vi "Conus_USB.vi"() -> ()   [LabVIEW 2017]
doc: "Conus USB - Versió bàsica de Conus / Sols adquisició i informe"
uses:
  Instance           2 17Saved   Conus_USB .vi
  Instance           1 17Saved   Conus_USB .vi
  Instance           4 17Saved   Conus_USB .vi
  <vilib>/DAQmx/write.llb/DAQmx Write (Digital 1D Bool NChan 1Samp 1Line).vi
  <vilib>/DAQmx/read.llb/DAQmx Read (Digital 1D Bool NChan 1Samp 1Line).vi
  Control 1.ctl
panel:
  out "Array":bool[](array[boolean])
  out "data":bool[](array[boolean])
  out "Fent_Rep":bool
  out "Booleans":refnum<vi>[](array[refnum])
  in  "Rep. Fetes":u8 caption="N. Rep."
  in  "Salir":bool caption="Sortir"
  in  "EtiquetaTipusParo":string caption="String"
  in  "Etiqueta Velocitats":string caption="String"
  out "appended array":refnum<vi>[](array[refnum])
  out "MissatgesUsuari":string[](array[string])
  out "Caselles":refnum<vi>[](array[refnum])
  out "StringsEstatMáquina":string[](array[string])
  in  "Rep. A Fer":sgl caption="N. Rep." format="%#_1g"
  out "ParoDefor":bool caption="ParoRotura"
  out "ParoDeforFet":bool caption="ParoProcessat"
  out "ParoCargaFet":bool caption="ParoProcessat"
  out "ParoCarga":bool caption="ParoProcessat"
  in  "CaptadorD":u16(ring) caption="Unidades" items=["Deformació", "Extensòmetre"]
  in  "FinalEnsayo":bool caption="Final prova"
  in  "ActivaParoCarga":bool caption="ActivaParoDefor"
  in  "ValorParoCarga":sgl caption="Força" min=0 format="%#.3f"
  in  "ActivaParoDefor":bool
  in  "ActivaParoRotura":T1
  in  "ValorParoDesplazamiento":sgl caption="Deformació" min=0 format="%#.3f"
  in  "ValorParoRotura":sgl caption="Ruptura (%)" min=0 format="%#_3f"
  out "Ensayo activo":bool caption="Prova en marxa"
  out "ArraiMostresxProva":dbl[](array[numeric])
  out "NMostres":dbl
  in  "BtEliminarUltima":bool=TRUE caption="Eliminar última prova"
  out "Estado ensayo:":string caption="Estat assaig:"
  out "CodiAturada":u32
  out "ViuMotor":bool
  out "MotorBipolar":bool
  out "Baixar":bool
  out "Pujar":bool
  out "PrimerCaptador":i32
  out "rings":refnum<vi>[](array[refnum])
  in  "IndexUnitatsD":u8
  in  "IndexUnitatsF":u8
  in  "IndexCaptadorD":u8
  in  "IndexCaptadorF":u8
  out "EtiquetesRegistre":string[](array[string])
  out "start":bool
  out "Active_motor":bool
  in  "Inici x Boto":bool
  out "ExtenPoten":bool caption="Extensòmetre Pot."
  out "ValorSenseTara":dbl
  in  "VelocitatMàxima":dbl
  in  "PerCentPrecarga":sgl=0.5 caption="Precàrrega (%)"
  in  "Precarga":bool
  in  "BtMaxF":bool
  in  "CaptadorF":u16(ring) caption="Unidades" items=["1000 kg"=11, "No presente"=23]
  in  "UnidadesF":u16(ring) caption="Unidades" items=["kg", "N"]
  in  "BtTaraF":bool caption="TARA"
  out "Fuerza":sgl caption="Força" format="%.1f"
  out "Nº Tests":u8 caption="Tests:"
  out "Sobrecarga":bool caption="Sobrecàrrega"
  out "Paro Manual":bool caption="Aturada Manual"
  out "FCI":bool
  out "FCS":bool
  in  "ResoExten":i8(ring) caption="Resolució Extensometre" items=["0.1", "0.2", "0.5", "0.01", "0.02", "0.05", "0.001", "0.002", "0.005"]
  out "PrecargaOn":bool
  in  "ValorPrecarga":dbl caption="Precarga (%)"
  out "Calibratge D":dbl[](array[numeric])
  out "Extensometre":bool
  in  "UnidadesD":u16(ring) caption="Unidades" items=["mm", "inch"]
  in  "BtTaraD":bool caption="TARA"
  out "Deformacion":sgl caption="Deformació" format="%.1f"
  out "Celula_0":u8
  in  "Células":u8(ring) caption="Célula 1" items=["0.5 kg", "1 Kg", "2 Kg", "5 kg", "10 kg", "20 kg", "50 kg", "100 kg", "200 kg", "300 kg", "500 kg", "1000 kg", "2000 kg", "5000 kg", "10000 kg", "20000 kg", "30000 kg", "P-20 kg", "P-200 kg", "P-500 kg", "P-5000 kg", "P-20000 kg", "P-50 bar", "No presente"]
  in  "UnidadesF_C2":u16(ring) caption="Unidades" items=["kg"]
  in  "UnidadesF_C1":u16(ring) caption="Unidades" items=["kg", "N"]
  out "ArraiUnitats":cluster{"String":string, "Value":u16}[](array[cluster])=[{"String"="kg", "Value"=0}, {"String"="N", "Value"=1}, {"String"="g", "Value"=2}, {"String"="daN", "Value"=3}, {"String"="cN", "Value"=4}, {"String"="KN", "Value"=5}, {"String"="lb", "Value"=6}]
  in  "UnitatsF":u8[](array[numeric])
  in  "Velocidad Retorno":sgl caption="Retorn" min=0 max=500 step=1 format="%#.1f"
  in  "Velocidad Ensayo":sgl caption="Assaig" min=0 step=1
  out "ValorSobrecargaC2":dbl
  out "Valor de control sobrecarga":dbl
  out "Calibratge":dbl[](array[numeric])
  in  "ParaAssaig":bool
  out "ParoProcessat":bool
  out "Salidas_mando":T2={"HI_down"=TRUE, " LO_down"=TRUE, "HI_up"=TRUE, "*"=TRUE, " LO_up"=TRUE, " start"=TRUE, " Ensayo_down"=TRUE, " Ensayo_up"=TRUE}
  out "VelocitatMotor":dbl min=0.0 max=500.0 step=1.0
  out "TempsLectura":u32=150
  out "Maxim":sgl
  in  "Inhibicio":bool
  in  "Ensayonuevo":bool caption="Assaig Nou"
  in  "Guardar":bool caption="Informe"
  in  "Iniciar / Finalizar":bool=TRUE caption="Finalitzar prova"
  out "TablaFinal":dbl[][](array[numeric])
  out "Tabla":dbl[][](array[numeric])
  in  "Columna":i32
  out "Paro Emergencia":bool
  out "ParoRotura":bool
  out "AssaigMM":bool
  out "DSenseTara":sgl caption="Fuerza - N"
  out "FactorsUnitatsPendents_D":dbl[](array[numeric])
  out "ConversioUnitatsD":dbl[](array[numeric])=[1.0, 9.8756, 1000.0, 0.98]
  in  "DadesAdquirides":dbl[](array[numeric]) format="%#_8g"
  out "FactorsUnitatsPendents_F":dbl[](array[numeric])
  in  "LedAssaig":bool
  out "BaixarMM":bool
  out "PujarMM":bool
  in  "TaraD":sgl
  in  "ValMax":bool
  out "FSenseTara":sgl caption="Fuerza - N"
  in  "TaraF":sgl
  out "Password":string
  out "ValorSobrecargaC1":dbl
  out "ConversioUnitatsF":dbl[](array[numeric])=[1.0, 9.8756, 2.2]
  out "Pendents":dbl[](array[numeric]) format="%#_8g"
  in  "Procesa datos":bool
  in  "Stop":bool=TRUE
  in  "First time":bool
  out "?":cluster{"Y":dbl[], "Y":dbl[]}[](graph)
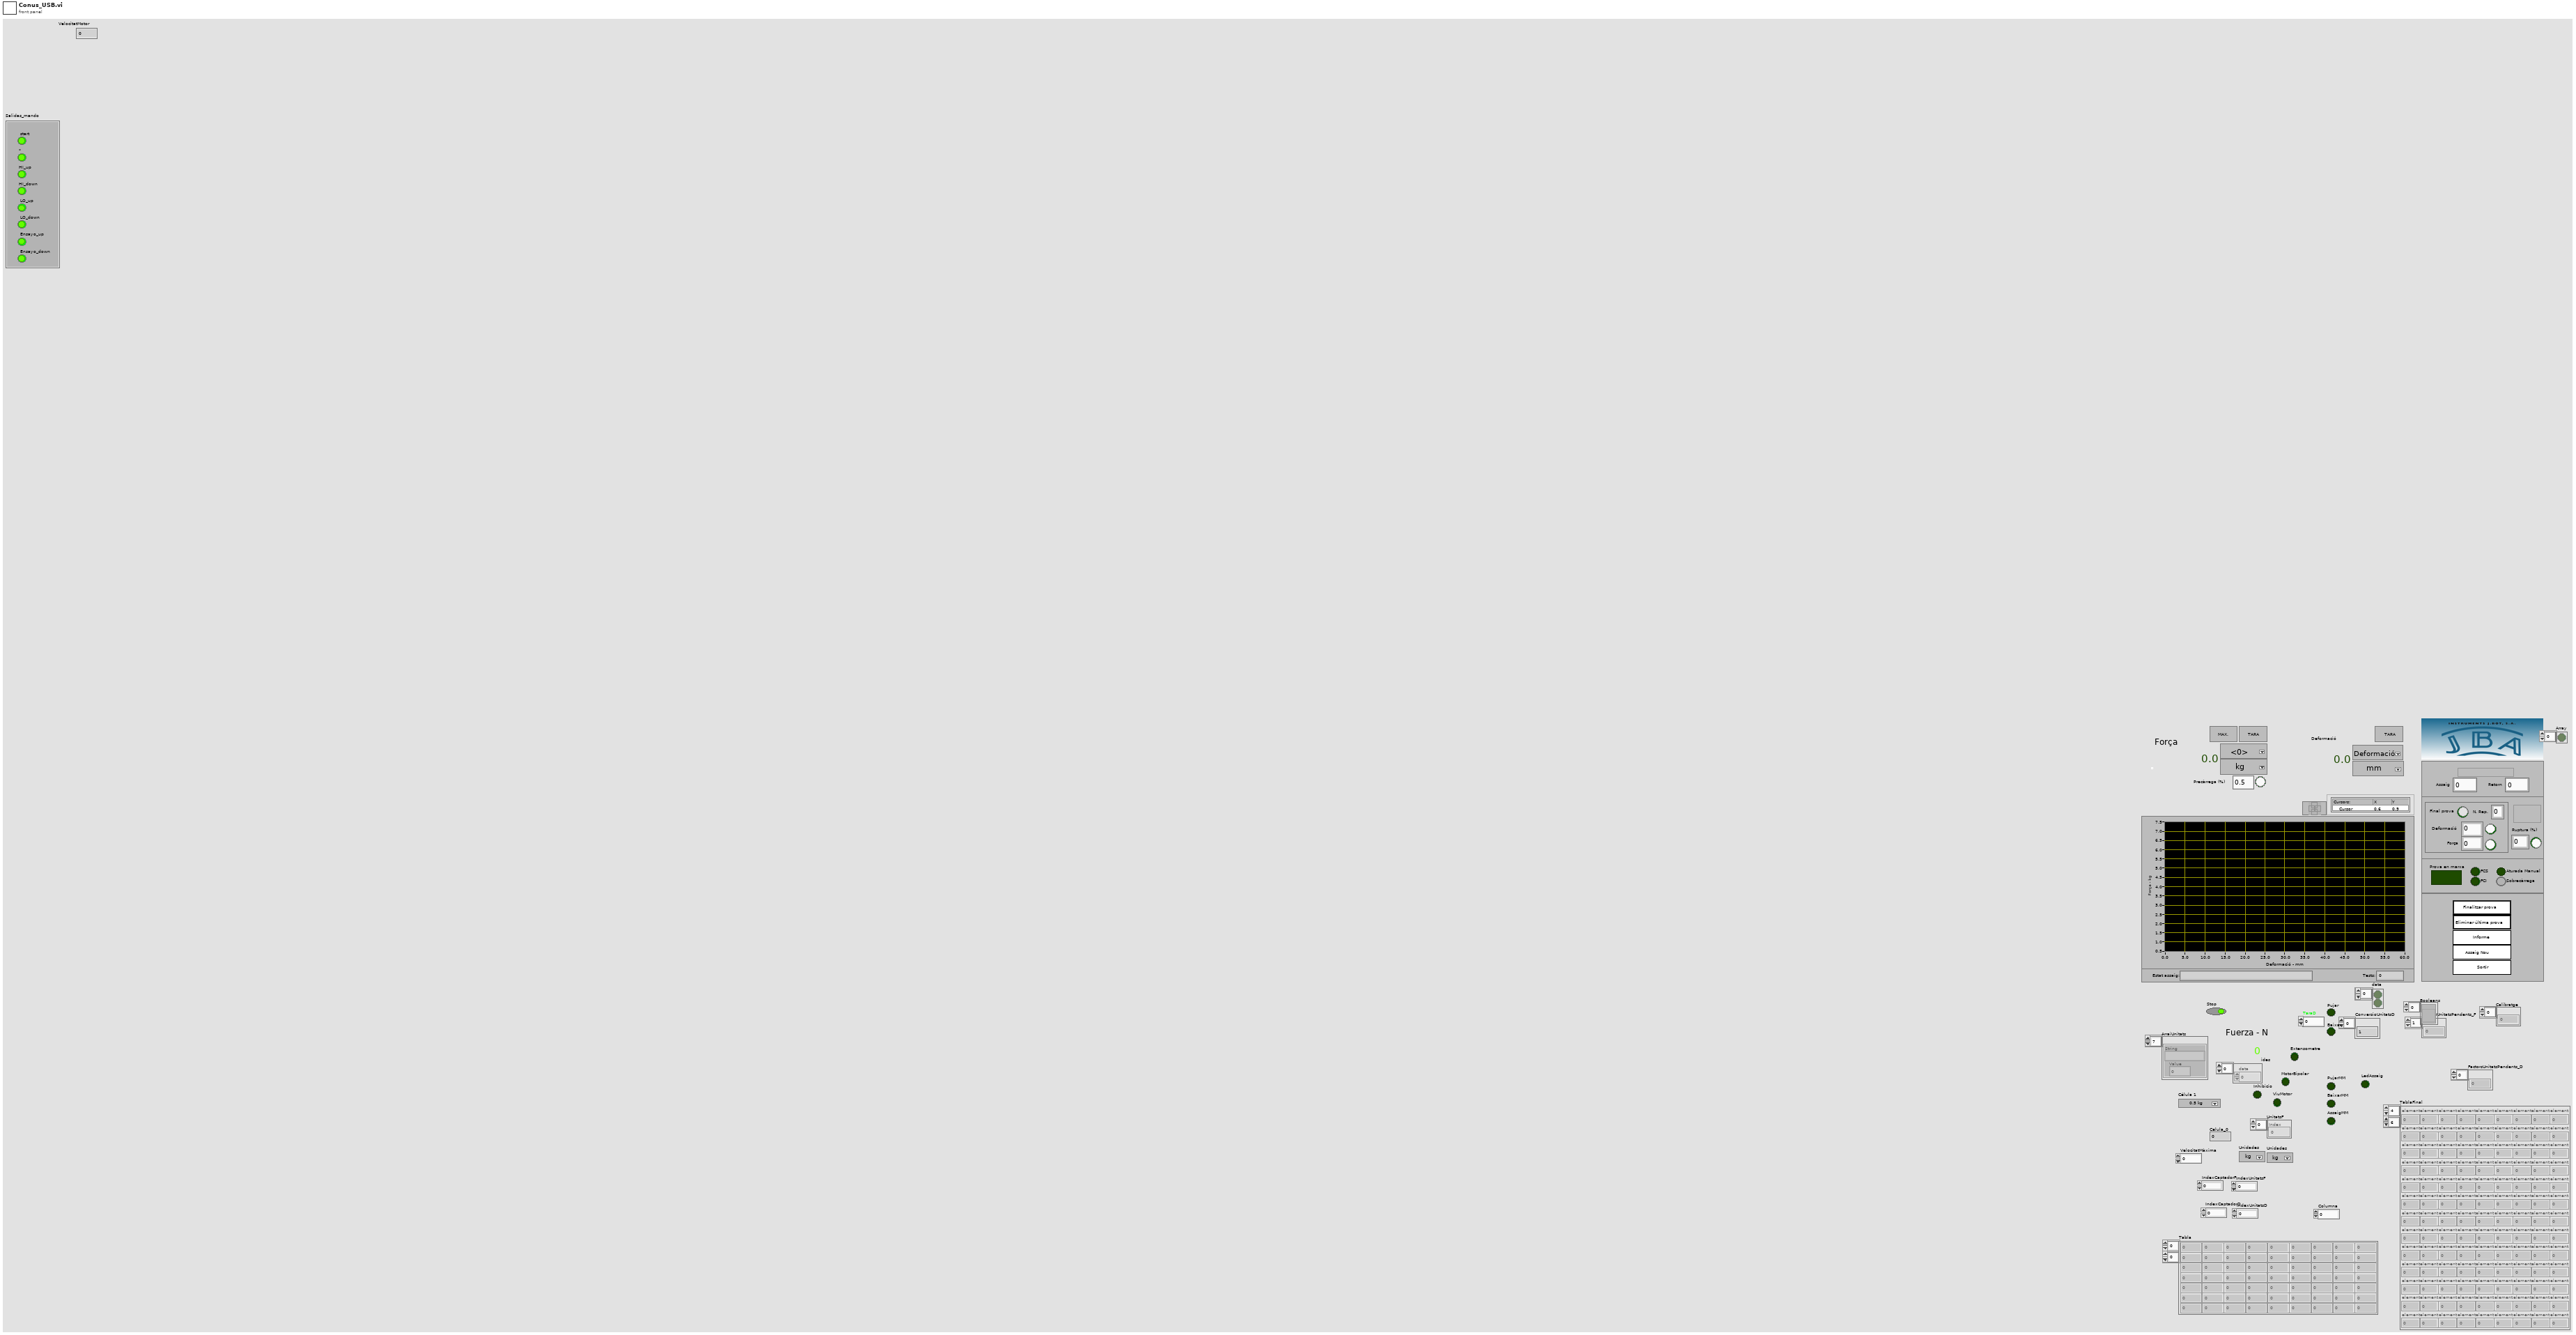
[diagram p1: front panel]
types:
  T1 = typedef "Control 1.ctl" = bool
  T2 = cluster{"HI_down":bool, " LO_down":bool, "HI_up":bool, "*":bool, " LO_up":bool, " start":bool, " Ensayo_down":bool, " Ensayo_up":bool}
  T3 = cluster{"HI_down":bool, "LO_down":bool, "HI_up":bool, "*":bool, "LO_up":bool, "start":bool, "Ensayo_down":bool, "Ensayo_up":bool}
  T4 = typedef "LVStringsAndValuesArrayTypeDef_U8.ctl" = cluster{"String":string, "Value":u8}[]
  T5 = cluster{"Boolean":bool, "element":bool, "Boolean":bool, "Boolean":bool}
  T6 = typedef "LVStringsAndValuesArrayTypeDef_U16.ctl" = cluster{"String":string, "Value":u16}[]
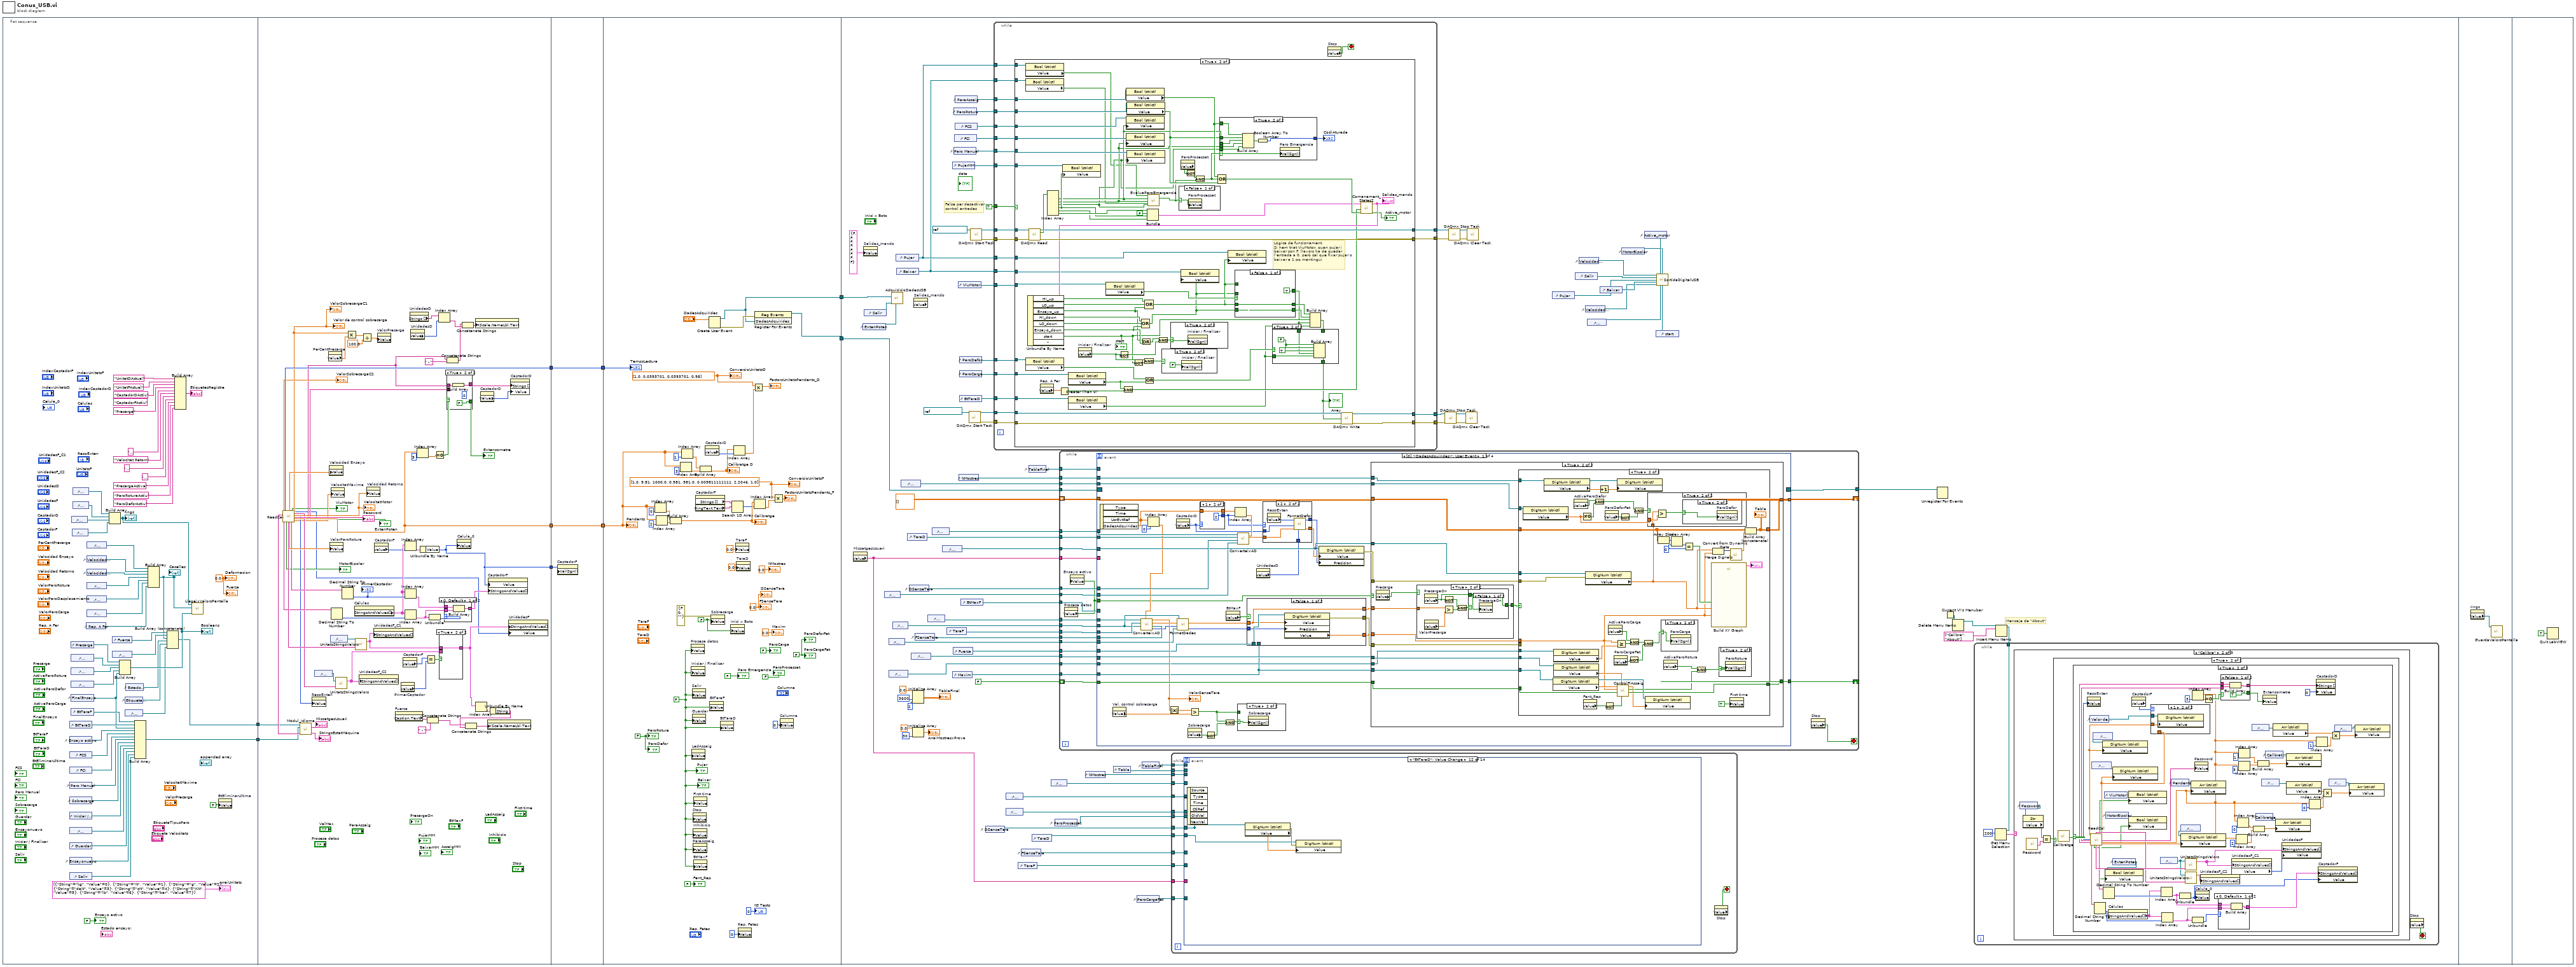
[diagram p0: block diagram]
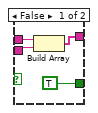
[diagram p3: hidden frame]
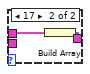
[diagram p4: hidden frame]
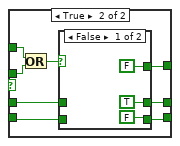
[diagram p7: hidden frame]
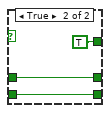
[diagram p8: hidden frame]
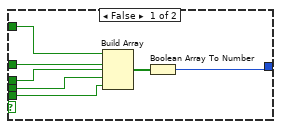
[diagram p11: hidden frame]
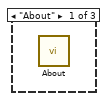
[diagram p13: hidden frame]
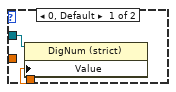
[diagram p16: hidden frame]
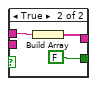
[diagram p17: hidden frame]
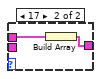
[diagram p18: hidden frame]
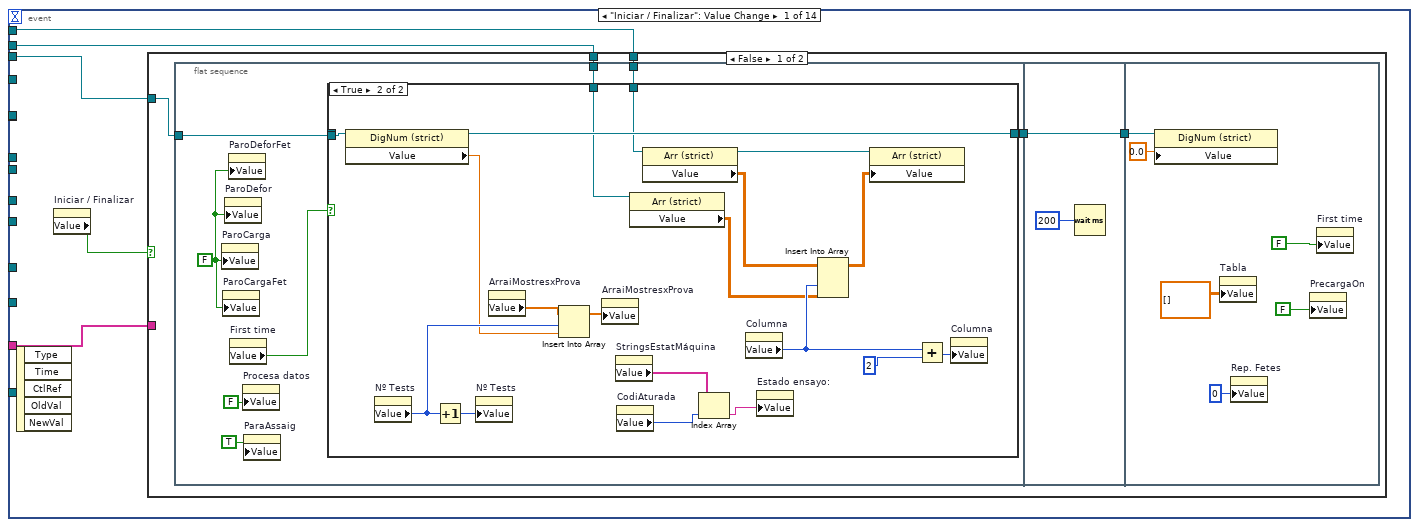
[diagram p20: hidden frame]
diagram:
  n1 = flat-sequence {
    tunnel: [w19] -> w2
    tunnel: [w18] -> w1
    tunnel: [w111] -> w9
    tunnel: [w126] -> w8
    tunnel: [w74] -> w3
    tunnel: w2 -> [w66]
    tunnel: w1 -> [w68]
    tunnel: w9 -> [w145]
    tunnel: [w145] -> w7
    tunnel: w8 -> [w144]
    tunnel: [w144] -> w6
    tunnel: w3 -> [w143]
    tunnel: w7 -> [w164]
    tunnel: [w183] -> w5
    tunnel: [w175] -> w4
    tunnel: w6 -> [w174]
    tunnel: w5 -> [w267]
    tunnel: w4 -> [w249]
    frame #0 {
      w12 = sgl 0.0 ("Deformacion")
      (unwired) "CaptadorFActiu" ("value")
      n2 = control-ref of="BtTaraD"() -> (w39:refnum<vi>)
      n3 = control-ref of="Ensayo activo"() -> (w37:refnum<vi>)
      n4 = control-ref of="FCS"() -> (w36:refnum<vi>)
      n5 = control-ref of="FCI"() -> (w35:refnum<vi>)
      n6 = control-ref of="Paro Manual"() -> (w34:refnum<vi>)
      n7 = control-ref of="Sobrecarga"() -> (w33:refnum<vi>)
      n8 = control-ref of="Iniciar / Finalizar"() -> (w32:refnum<vi>)
      n9 = control-ref of="BtEliminarUltima"() -> (w31:refnum<vi>)
      n10 = control-ref of="Guardar"() -> (w17:refnum<vi>)
      n11 = control-ref of="Ensayonuevo"() -> (w30:refnum<vi>)
      n12 = control-ref of="Salir"() -> (w29:refnum<vi>)
      n13 = control-ref of="Precarga"() -> (w50:refnum<vi>)
      n14 = control-ref of="ActivaParoRotura"() -> (w49:refnum<vi>)
      n15 = control-ref of="ActivaParoDefor"() -> (w48:refnum<vi>)
      n16 = control-ref of="ActivaParoCarga"() -> (w42:refnum<vi>)
      n17 = control-ref of="FinalEnsayo"() -> (w38:refnum<vi>)
      n18 = control-ref of="BtTaraF"() -> (w40:refnum<vi>)
      n19 = control-ref of="CaptadorD"() -> (w45:refnum<vi>)
      n20 = control-ref of="CaptadorF"() -> (w44:refnum<vi>)
      n21 = control-ref of="UnidadesD"() -> (w47:refnum<vi>)
      n22 = control-ref of="UnidadesF"() -> (w46:refnum<vi>)
      n23 = control-ref of="Rep. A Fer"() -> (w10:refnum<vi>)
      n24 = control-ref of="PerCentPrecarga"() -> (w27:refnum<vi>)
      n25 = control-ref of="Velocidad Ensayo"() -> (w26:refnum<vi>)
      n26 = control-ref of="Velocidad Retorno"() -> (w51:refnum<vi>)
      n27 = control-ref of="ValorParoRotura"() -> (w25:refnum<vi>)
      n28 = control-ref of="ValorParoDesplazamiento"() -> (w24:refnum<vi>)
      n29 = control-ref of="ValorParoCarga"() -> (w23:refnum<vi>)
      n30 = Build Array(w47, w46, w45, w44) -> (w43:refnum<vi>[])
      "rings" <- w43
      n31 = control-ref of="Fuerza"() -> (w22:refnum<vi>)
      n32 = control-ref of="Deformacion"() -> (w21:refnum<vi>)
      n33 = Build Array(w50, w49, w48, w42, w38) -> (w28:refnum<vi>[])
      "Booleans" <- w28
      n34 = control-ref of="Etiqueta Velocitats"() -> (w14:refnum<vi>)
      n35 = control-ref of="EtiquetaTipusParo"() -> (w13:refnum<vi>)
      n36 = control-ref of="Estado ensayo:"() -> (w15:refnum<vi>)
      n37 = Build Array(w40, w39, w38, w37, w36, w35, w34, w33, w32, w31, w17, w30, w29) -> (w19:refnum<vi>[])
      n38 = Build Array(w27, w26, w51, w25, w24, w23, w10) -> (w16:refnum<vi>[])
      "Caselles" <- w16
      n39 = Build Array (concatenate)(w22, w21, w16, w15, w14, w13) -> (w18:refnum<vi>[])
      n40 = Build Array("UnitatDActual" ("value"), "UnitatFActual" ("value"), "CaptadorDActiu" ("value"), "Precarga" ("value"), "Velocitat" ("value"), "Velocitat Retorn" ("value"), "Rotura" ("value"), "Desplazamiento" ("value"), "PrecargaActiva" ("value"), "ParoRoturaActiu" ("value"), "ParoDeforActiu" ("value")) -> (→"EtiquetesRegistre":string[])
      n41 = call "LlegeixValorsPantalla.vi"("rings"=w43, "Caselles 2"=w16, "Booleans"=w28) -> ()  [unwired: 8 in]
      n42 = property on="BtEliminarUltima" class="Bool (strict)"("Value"=FALSE ("BtEliminarUltima")) -> ()  [unwired: 2 in, 2 out]
      "Ensayo activo" <- FALSE ("Ensayo activo")
      "Fuerza" <- w12
      "Deformacion" <- w12
      "ArraiUnitats" <- cluster{"String":string, "Value":u16}[] [{"String"="kg", "Value"=0}, {"String"="N", "Value"=1}, {"String"="g", "Value"=2}, {"String"="daN", "Value"=3}, {"String"="cN", "Value"=4}, {"String"="KN", "Value"=5}, {"String"="lb", "Value"=6}, {"String"="bar", "Value"=7}] ("Strings And Values [] 2")
    }
    frame #1 {
      n43 = call "ReadCal.vi"() -> ("SobrecargaC2"=→"ValorSobrecargaC2":dbl, "ResoExten"=w103:i8, "TextExtensometre"=w108:string, "TextDeformacio"=w67:string, "SegonCaptador"=w118:string, "TempsLectura"=w126:u16, "Idioma"=w70:string, "MotorBipolar"=→"MotorBipolar":bool, "UnitatsC2"=w119:string, "UnitatsC1"=w120:string, "Velocitat"=w127:dbl, "ParoRotura"=w128:dbl, "V. Retorn"=w123:dbl, "PrimerCaptador"=w116:string, "ViuMotor"=→"ViuMotor":bool, "ExtenPoten"=→"ExtenPoten":bool, "Unidades"=w64:u8, "SobrecargaC1"=w104:dbl, "Password"=→"Password":string, "Pendents"=w111:dbl[], "VelocitatMàxima"=w100:dbl)  [unwired: 4 in, 3 out]
      "VelocitatMotor" <- w123
      "ValorSobrecargaC1" <- w104
      "Valor de control sobrecarga" <- w104
      n44 = call "Módul_Idioma.vi"("Idioma"=w70, "Array"=w66, "Caselles"=w68) -> ("TextosEstatMaquina"=→"StringsEstatMáquina":string[], "MissatgesUsuari"=→"MissatgesUsuari":string[])  [unwired: 7 in]
      n45 = property on="ResoExten" class="Ring (strict)"("Value"=w103) -> ()  [unwired: 2 in, 2 out]
      n46 = control-ref of="ArraiUnitats"() -> (w121:refnum<vi>)
      n47 = property on="PerCentPrecarga" class="DigNum (strict)"() -> ("Value"=w94:sgl)  [unwired: 2 in, 2 out]
      n48 = property on="Velocidad Ensayo" class="DigNum (strict)"("Value"=w127) -> ()  [unwired: 2 in, 2 out]
      n49 = property on="ValorParoRotura" class="DigNum (strict)"("Value"=w128) -> ()  [unwired: 2 in, 2 out]
      n50 = control-ref of="ArraiUnitats"() -> (w122:refnum<vi>)
      n51 = property on="VelocitatMàxima" class="DigNum (strict)"("Value"=w100) -> ()  [unwired: 2 in, 2 out]
      n52 = Decimal String To Number(string=w118) -> (number=w117:i32)  [unwired: 2 in, 1 out]
      n53 = call "UnitatsStringsValors.vi"("UnitatsC1"=w119, "Arr Refnum"=w121) -> ("Array 2"=w84:cluster{"String":string, "Value":u16}[])  [unwired: 1 out]
      n54 = Decimal String To Number(string=w116) -> (number=w115:i32)  [unwired: 2 in, 1 out]
      "PrimerCaptador" <- w115
      n55 = Multiply(x=w104, y=w94) -> (x*y=w106:dbl)
      n56 = property on="Células" class="Ring (strict)"() -> ("StringsAndValues[]"=w91:T4)  [unwired: 2 in, 2 out]
      n57 = call "UnitatsStringsValors.vi"("UnitatsC1"=w120, "Arr Refnum"=w122) -> ("Array 2"=w85:cluster{"String":string, "Value":u16}[])  [unwired: 1 out]
      n58 = property on="UnidadesF_C2" class="Ring (strict)"("StringsAndValues[]"=w84) -> ()  [unwired: 2 in, 2 out]
      n59 = Divide(x=w106, y=100.0) -> (x/y=w101:dbl)
      n60 = property on="Velocidad Retorno" class="DigNum (strict)"("Value"=w123) -> ()  [unwired: 2 in, 2 out]
      n61 = property on="UnidadesF_C1" class="Ring (strict)"("StringsAndValues[]"=w85) -> ()  [unwired: 2 in, 2 out]
      n62 = property on="CaptadorF" class="Ring (strict)"() -> ("Value"=w89:u16)  [unwired: 2 in, 2 out]
      n63 = property on="ValorPrecarga" class="DigNum (strict)"("Value"=w101) -> ()  [unwired: 2 in, 2 out]
      n64 = property on="Fuerza" class="DigNum (strict)"() -> ("Caption.Text"=w97:string)  [unwired: 2 in, 2 out]
      n65 = property on="PrimerCaptador" class="DigNum (strict)"() -> ("Value"=w86:i32)  [unwired: 2 in, 2 out]
      n66 = property on="CaptadorF" class="Ring (strict)"() -> ("Value"=w87:u16)  [unwired: 2 in, 2 out]
      n67 = Index Array(array=w91, index=w89) -> (element=w90:cluster{"String":string, "Value":u8})
      n68 = Index Array(array=w91, index=w115) -> (element=w93:cluster{"String":string, "Value":u8})
      n69 = Index Array(array=w91, index=w117) -> (element=w113:cluster{"String":string, "Value":u8})
      n70 = property on="UnidadesD" class="Ring (strict)"() -> ("Strings []"=w79:string[])  [unwired: 2 in, 2 out]
      n71 = property on="UnidadesD" class="Ring (strict)"() -> ("Value"=w78:u16)  [unwired: 2 in, 2 out]
      n72 = Index Array(array=w111, index=3) -> (element=w109:dbl)
      n73 = Unbundle By Name(w90) -> ("Value"=w74:u8)
      n74 = Equal?(x=w87, y=w86) -> (x = y?=w88:bool)
      n75 = Concatenate Strings(w97, " - ") -> (w96:string)
      n76 = Unbundle(w113) -> ("Value"=w114:u8)  [unwired: 1 out]
      n77 = Equal To 0?(x=w109) -> (x = 0?=w112:bool)
      n78 = Index Array(array=w79, index=w78) -> (element=w77:string)
      n79 = case shown="True" w88 {
        tunnel: w85 -> [_ w130]
        tunnel: [w129 w130] -> w65
        tunnel: w84 -> [w129 _]
        frame False {
        }
        frame True {
        }
      }
      n80 = case shown="0, Default" w114 {
        tunnel: w93 -> [w140 w141]
        tunnel: w113 -> [w139 _]
        tunnel: [w138 w142] -> w92
        frame 0, Default {
          n81 = Build Array(w140, w139) -> (w138:cluster{"String":string, "Value":u8}[])
        }
        frame 17 {
          n82 = Build Array(w141) -> (w142:cluster{"String":string, "Value":u8}[])
        }
      }
      n83 = Concatenate Strings(w67, " - ") -> (w75:string)
      n84 = case shown="True" w112 {
        tunnel: w108 -> [w134 _]
        tunnel: [w133 w135] -> w80
        tunnel: [TRUE ("Extensometre") FALSE ("Extensometre")] -> w107
        tunnel: w67 -> [w131 w136]
        frame False {
          n85 = Build Array(w131, w134) -> (w133:string[])
        }
        frame True {
          (unwired) 0 ("index")
          n86 = Build Array(w136) -> (w135:string[])
        }
      }
      "Extensometre" <- w107
      n87 = property on="Celula_0" class="DigNum (strict)"("Value"=w74) -> ()  [unwired: 2 in, 2 out]
      n88 = Concatenate Strings(w75, w77) -> (w95:string)
      n89 = property class="XYGraph (strict)"("XScale.NameLbl.Text"=w95) -> ()  [unwired: 2 in, 2 out]
      n90 = Index Array(array=w65) -> (element=w82:cluster{"String":string, "Value":u16})  [unwired: 1 in]
      n91 = property on="CaptadorD" class="Ring (strict)"() -> ("Value"=w81:u16)  [unwired: 2 in, 2 out]
      n92 = property on="CaptadorF" class="Ring (strict)"("Value"=w74, "StringsAndValues[]"=w92) -> ()  [unwired: 2 in, 2 out]
      n93 = Unbundle By Name(w82) -> ("String"=w83:string)
      n94 = Concatenate Strings(w96, w83) -> (w102:string)
      n95 = property class="XYGraph (strict)"("YScale.NameLbl.Text"=w102) -> ()  [unwired: 2 in, 2 out]
      n96 = property on="UnidadesF" class="Ring (strict)"("StringsAndValues[]"=w65, "Value"=w64) -> ()  [unwired: 2 in, 2 out]
      n97 = property on="CaptadorD" class="Ring (strict)"("Strings []"=w80, "Value"=w81) -> ()  [unwired: 2 in, 2 out]
    }
    frame #2 {
      n98 = property on="CaptadorF" class="Ring (strict)"("Val(Sgnl)"=w143) -> ()  [unwired: 2 in, 2 out]
    }
    frame #3 {
      w149 = FALSE ("ParoCargaFet")
      w148 = FALSE ("ParoRotura")
      w162 = dbl[] [1.0, 0.0393701, 0.0393701, 0.98]
      w177 = sgl 0.0 ("FSenseTara")
      w185 = dbl[] [1.0, 9.81, 1000.0, 0.981, 981.0, 0.009811111111, 2.2046, 1.0]
      w156 = FALSE ("Sobrecarga")
      w152 = FALSE ("Iniciar / Finalizar")
      n99 = Index Array(array=w164, index=0) -> (element=w170:dbl)
      n100 = Index Array(array=w164, index=2) -> (element=w171:dbl)
      n101 = Build Array(w170, w171) -> (w169:dbl[])
      "Calibratge" <- w169
      n102 = Index Array(array=w164, index=3) -> (element=w165:dbl)
      n103 = Index Array(array=w164, index=1) -> (element=w163:dbl)
      n104 = property on="Procesa datos" class="Bool (strict)"("Value"=w152) -> ()  [unwired: 2 in, 2 out]
      n105 = property on="Iniciar / Finalizar" class="Bool (strict)"("Value"=w152) -> ()  [unwired: 2 in, 2 out]
      n106 = property on="LedAssaig" class="Bool (strict)"("Value"=w152) -> ()  [unwired: 2 in, 2 out]
      n107 = property on="Salir" class="Bool (strict)"("Value"=w152) -> ()  [unwired: 2 in, 2 out]
      n108 = property on="Guardar" class="Bool (strict)"("Value"=w152) -> ()  [unwired: 2 in, 2 out]
      n109 = property on="Stop" class="Bool (strict)"("Value"=w152) -> ()  [unwired: 2 in, 2 out]
      n110 = property on="Inhibicio" class="Bool (strict)"("Value"=w152) -> ()  [unwired: 2 in, 2 out]
      n111 = property on="ParaAssaig" class="Bool (strict)"("Value"=w152) -> ()  [unwired: 2 in, 2 out]
      n112 = property on="First time" class="Bool (strict)"("Value"=w152) -> ()  [unwired: 2 in, 2 out]
      n113 = property on="BtMaxF" class="Bool (strict)"("Value"=w152) -> ()  [unwired: 2 in, 2 out]
      n114 = property on="CaptadorF" class="Ring (strict)"() -> ("Strings []"=w155:string[], "RingText.Text"=w154:string)  [unwired: 2 in, 2 out]
      n115 = Build Array(w163, w165) -> (w160:dbl[])
      "Calibratge D" <- w160
      n116 = property on="CaptadorD" class="Ring (strict)"() -> ("Value"=w161:u16)  [unwired: 2 in, 2 out]
      n117 = Create User Event(user event datatype="DadesAdquirides") -> (user event=w175:refnum<user-event>, error out=w182:errorcluster)  [unwired: 1 in]
      n118 = property on="BtTaraF" class="Bool (strict)"("Value"=w152) -> ()  [unwired: 2 in, 2 out]
      n119 = property on="Sobrecarga" class="Bool (strict)"(error in=errorcluster {"status"=FALSE, "code"=0, "source"=""} ("error in (no error)"), "Value"=w156) -> ()  [unwired: 1 in, 2 out]
      n120 = property on="BtTaraD" class="Bool (strict)"("Value"=w152) -> ()  [unwired: 2 in, 2 out]
      n121 = property on="Inici x Boto" class="Bool (strict)"("Value"=w156) -> ()  [unwired: 2 in, 2 out]
      n122 = Search 1D Array(1D array=w155, element=w154) -> (index of element=w153:i32)  [unwired: 1 in]
      n123 = Index Array(array=w160, index=w161) -> (element=w159:dbl)
      n124 = property on="TaraF" class="DigNum (strict)"("Value"=sgl 0.0 ("Tara")) -> ()  [unwired: 2 in, 2 out]
      n125 = property on="TaraD" class="DigNum (strict)"("Value"=sgl 0.0 ("TaraD")) -> ()  [unwired: 2 in, 2 out]
      n126 = property on="Rep. Fetes" class="DigNum (strict)"("Value"=u8 0 ("Rep. Fetes")) -> ()  [unwired: 2 in, 2 out]
      n127 = Multiply(x=w162, y=w159) -> (x*y=→"FactorsUnitatsPendents_D":dbl[])
      n128 = Index Array(array=w169, index=w153) -> (element=w168:dbl)
      n129 = register-events(error in=w182, w175) -> (reference out=w183:refnum<event-registration>)  [unwired: 1 in, 1 out]
      n130 = Multiply(x=w185, y=w168) -> (x*y=→"FactorsUnitatsPendents_F":dbl[])
      n131 = property on="Columna" class="DigNum (strict)"("Value"=0 ("Columna")) -> ()  [unwired: 2 in, 2 out]
      "Pendents" <- w164
      "ConversioUnitatsF" <- w185
      "FSenseTara" <- w177
      "ConversioUnitatsD" <- w162
      "DSenseTara" <- w177
      "ParoRotura" <- w148
      "Paro Emergencia" <- FALSE ("Paro Emergencia")
      "Maxim" <- sgl 0.0 ("Maxim")
      "TempsLectura" <- w174
      "ParoProcessat" <- FALSE ("ParoProcessat")
      "Nº Tests" <- u8 0 ("Nº Tests")
      "Pujar" <- w152
      "Baixar" <- w152
      "NMostres" <- 0.0 ("NMostres")
      "ParoCarga" <- FALSE ("ValorCargaFet")
      "ParoCargaFet" <- w149
      "ParoDeforFet" <- w149
      "ParoDefor" <- w148
      "Fent_Rep" <- FALSE ("Fent_Rep")
    }
    frame #4 {
      # "False per desactivar\ncontrol entrades"
      # "Mensaje de \"About\""
      n132 = property on="MissatgesUsuari" class="Arr (strict)"() -> ("Value"=w195:string[])  [unwired: 2 in, 2 out]
      n133 = control-ref of="ExtenPoten"() -> (w216:refnum<vi>)
      n134 = property on="Salidas_mando" class="Clust (strict)"("Value"=T3 {"HI_down"=FALSE, "LO_down"=FALSE, "HI_up"=FALSE, "*"=FALSE, "LO_up"=FALSE, "start"=FALSE, "Ensayo_down"=FALSE, "Ensayo_up"=FALSE} ("Salidas_mando")) -> ()  [unwired: 2 in, 2 out]
      n135 = control-ref of="Salir"() -> (w250:refnum<vi>)
      n136 = control-ref of="UnidadesD"() -> (w260:refnum<vi>)
      n137 = control-ref of="ValorParoCarga"() -> (w200:refnum<vi>)
      n138 = control-ref of="CaptadorF"() -> (w225:refnum<vi>)
      n139 = call "AdquisicioDadesUSB.vi"(6:w216, "Stop"=w250, 10:w249) -> ()  [unwired: 9 in]
      n140 = control-ref of="UnidadesF"() -> (w259:refnum<vi>)
      n141 = control-ref of="Pujar"() -> (w206:refnum<vi>)
      n142 = control-ref of="Baixar"() -> (w205:refnum<vi>)
      n143 = control-ref of="ValorParoDesplazamiento"() -> (w221:refnum<vi>)
      n144 = control-ref of="TaraD"() -> (w263:refnum<vi>)
      n145 = control-ref of="DSenseTara"() -> (w264:refnum<vi>)
      n146 = control-ref of="ValorParoRotura"() -> (w256:refnum<vi>)
      n147 = Initialize Array(0.0 ("element"), 3600 ("dimension size"), 2 ("dimension size")) -> (→"TablaFinal":dbl[][])
      n148 = Initialize Array(0.0 ("element"), 30 ("dimension size")) -> (→"ArraiMostresxProva":dbl[])
      n149 = property on="Salidas_mando" class="Clust (strict)" props=["Value"]() -> ()  [unwired: 2 in, 3 out]
      n150 = control-ref of="FSenseTara"() -> (w269:refnum<vi>)
      n151 = control-ref of="FactorsUnitatsPendents_F"() -> (w268:refnum<vi>)
      n152 = control-ref of="FactorsUnitatsPendents_D"() -> (w266:refnum<vi>)
      n153 = control-ref of="Deformacion"() -> (w265:refnum<vi>)
      n154 = control-ref of="TaraF"() -> (w270:refnum<vi>)
      n155 = control-ref of="PujarMM"() -> (w208:refnum<vi>)
      n156 = control-ref of="Maxim"() -> (w248:refnum<vi>)
      n157 = control-ref of="Fuerza"() -> (w218:refnum<vi>)
      n158 = control-ref of="Paro Manual"() -> (w229:refnum<vi>)
      n159 = control-ref of="ParoRotura"() -> (w228:refnum<vi>)
      n160 = control-ref of="FCI"() -> (w230:refnum<vi>)
      n161 = control-ref of="ParaAssaig"() -> (w227:refnum<vi>)
      n162 = control-ref of="FCS"() -> (w231:refnum<vi>)
      n163 = control-ref of="ViuMotor"() -> (w209:refnum<vi>)
      n164 = control-ref of="NMostres"() -> (w201:refnum<vi>)
      n165 = control-ref of="ParoDefor"() -> (w198:refnum<vi>)
      n166 = control-ref of="ParoCarga"() -> (w199:refnum<vi>)
      n167 = control-ref of="BtTaraD"() -> (w193:refnum<vi>)
      n168 = control-ref of="BtMaxF"() -> (w223:refnum<vi>)
      n169 = call <vilib>:"DAQmx Start Task.vi"("task/channels in"=refnum<k21> "USBDigitalOut") -> ("task out"=w237:refnum<k21>, "error out"=w236:errorcluster)  [unwired: 13 in]
      n170 = call <vilib>:"DAQmx Start Task.vi"("task/channels in"=refnum<k21> "USBDigitalIn") -> ("task out"=w245:refnum<k21>, "error out"=w244:errorcluster)  [unwired: 13 in]
      n171 = control-ref of="DSenseTara"() -> (w261:refnum<vi>)
      n172 = while {
        tunnel: w245 -> [w298]
        tunnel: w244 -> [w297]
        tunnel: [w296] -> w240
        tunnel: [w295] -> w239
        tunnel: w237 -> [w294]
        tunnel: w236 -> [w293]
        tunnel: [w292] -> w233
        tunnel: [w291] -> w232
        tunnel: w231 -> [w290]
        tunnel: w230 -> [w289]
        tunnel: w229 -> [w288]
        tunnel: w228 -> [w287]
        tunnel: w227 -> [w286]
        tunnel: TRUE -> [w285]
        tunnel: w206 -> [w283]
        tunnel: w205 -> [w282]
        tunnel: w209 -> [w281]
        tunnel: w208 -> [w280]
        tunnel: w205 -> [w279]
        tunnel: w206 -> [w278]
        tunnel: w199 -> [w277]
        tunnel: w198 -> [w276]
        tunnel: w193 -> [w275]
        stop <- w284 stop-if-true
        n173 = case shown="True" w285 {
          tunnel: w298 -> [w302 w373]
          tunnel: w297 -> [w301 w372]
          tunnel: [w302 w371] -> w296
          tunnel: [w301 w370] -> w295
          tunnel: w294 -> [w300 w365]
          tunnel: w293 -> [w299 w364]
          tunnel: [w299 w363] -> w292
          tunnel: [w300 w362] -> w291
          tunnel: w290 -> [_ w359]
          tunnel: w289 -> [_ w358]
          tunnel: w288 -> [_ w357]
          tunnel: w287 -> [_ w350]
          tunnel: w286 -> [_ w347]
          tunnel: w283 -> [_ w340]
          tunnel: w282 -> [_ w339]
          tunnel: w281 -> [_ w337]
          tunnel: w280 -> [_ w327]
          tunnel: w279 -> [_ w324]
          tunnel: w278 -> [_ w323]
          tunnel: w277 -> [_ w314]
          tunnel: w276 -> [_ w313]
          tunnel: w275 -> [_ w305]
          frame False {
          }
          frame True {
            # "Lògica de funcionament.\nSi hem triat ViuMotor, quan pujar i baixar son F, llavors ha de quedar l'entrada a 0, però cal que fixar pujar o baixar a 1 pq mantingui"
            n174 = property class="Bool (strict)"(reference=w324) -> ("Value"=w317:bool)  [unwired: 1 in, 2 out]
            n175 = property class="Bool (strict)"(reference=w313) -> ("Value"=w312:bool)  [unwired: 1 in, 2 out]
            n176 = property class="Bool (strict)"(reference=w323) -> ("Value"=w318:bool)  [unwired: 1 in, 2 out]
            n177 = call-poly <vilib>:"DAQmx Read.vi"("task/channels in"=w373, "error in"=w372) -> ("task out"=w371:refnum<k21>, "data"=w331:bool[], "error out"=w370:errorcluster)  [unwired: 11 in]
            n178 = property on="Rep. A Fer" class="DigNum (strict)"() -> ("Value"=w309:sgl)  [unwired: 2 in, 2 out]
            n179 = Index Array(array=w331) -> (element #1=w321:bool, element #2=w320:bool, element #3=w319:bool, element #4=w325:bool, element #5=w326:bool, element #6=w361:bool)  [unwired: 6 in]
            n180 = Greater Than 0?(x=w309) -> (x > 0?=w307:bool)
            n181 = property class="Bool (strict)"(reference=w327, "Value"=w325) -> ()  [unwired: 1 in, 2 out]
            n182 = property class="Bool (strict)"(reference=w314) -> ("Value"=w308:bool)  [unwired: 1 in, 2 out]
            n183 = property class="Bool (strict)"(reference=w305) -> ("Value"=w303:bool)  [unwired: 1 in, 2 out]
            n184 = property on="Iniciar / Finalizar" class="Bool (strict)"() -> ("Value"=w344:bool)  [unwired: 2 in, 2 out]
            n185 = property class="Bool (strict)"(reference=w337) -> ("Value"=w336:bool)  [unwired: 1 in, 2 out]
            n186 = Not(x=w344) -> (.not. x?=w352:bool)
            n187 = And(x=w308, y=w307) -> (x .and. y?=w306:bool)
            n188 = property class="Bool (strict)"(reference=w347) -> ("Value"=w330:bool)  [unwired: 1 in, 2 out]
            n189 = property class="Bool (strict)"(reference=w359, "Value"=w321) -> ()  [unwired: 1 in, 2 out]
            n190 = property class="Bool (strict)"(reference=w358, "Value"=w320) -> ()  [unwired: 1 in, 2 out]
            n191 = property class="Bool (strict)"(reference=w350) -> ("Value"=w329:bool)  [unwired: 1 in, 2 out]
            n192 = property class="Bool (strict)"(reference=w357, "Value"=w319) -> ()  [unwired: 1 in, 2 out]
            n193 = Or(x=w312, y=w308) -> (x .or. y?=w311:bool)
            n194 = Bundle("Boolean"=w361, "element"=FALSE, "Boolean"=w325, "Boolean"=w326) -> (w310:T5)  [unwired: 1 in]
            n195 = call "EvaluaParoEmergencia.vi"("EsticPujant"=w318, "FCI"=w320, "FCS"=w321, "EsticBaixant"=w317, "ParoManual"=w319) -> ("Paro"=w322:bool)  [unwired: 10 in]
            n196 = case shown="False" w322 {
              selector: w322 -> [w398 _]
              frame False {
                n197 = property on="ParoProcessat" class="Bool (strict)"("Value"=w398) -> ()  [unwired: 2 in, 2 out]
              }
              frame True {
              }
            }
            n198 = property on="ParoProcessat" class="Bool (strict)"() -> ("Value"=w349:bool)  [unwired: 2 in, 2 out]
            n199 = Not(x=w349) -> (.not. x?=w348:bool)
            n200 = And(x=w348, y=w322) -> (x .and. y?=w346:bool)
            n201 = Compound Arithmetic op=OR(w330, w346, w329) -> (w345:bool)
            n202 = case shown="True" w346 {
              selector: w346 -> [_ w413]
              tunnel: w330 -> [w404 w412]
              tunnel: w329 -> [w403 w411]
              tunnel: w321 -> [w402 w410]
              tunnel: w320 -> [w401 w409]
              tunnel: w319 -> [w400 w408]
              tunnel: [w399 w406] -> w328
              frame False {
                n203 = Build Array(w404, w403, w402, w401, w400) -> (w405:bool[])
                n204 = Boolean Array To Number(Boolean array=w405) -> (number=w399:u32)
              }
              frame True {
                n205 = Build Array(w412, w411, w410, w409, w408) -> (w407:bool[])
                n206 = Boolean Array To Number(Boolean array=w407) -> (number=w406:u32)
                n207 = property on="Paro Emergencia" class="Bool (strict)"("Val(Sgnl)"=w413) -> ()  [unwired: 2 in, 2 out]
              }
            }
            "CodiAturada" <- w328
            n208 = call "Comanament_States2.vi"("Emergencia"=w345, "ReseUpDown"=w306, "Entradas_Botones"=w310) -> ("Active_motor"=→"Active_motor":bool, "Salidas_mando"=w351:T2)  [unwired: 5 in]
            "Salidas_mando" <- w351
            n209 = Unbundle By Name(w351) -> ("HI_up"=w369:bool, "LO_up"=w368:bool, "Ensayo_up"=w355:bool, "HI_down"=w367:bool, "LO_down"=w366:bool, "Ensayo_down"=w356:bool, "start"=w338:bool)  [unwired: 1 out]
            "start" <- w338
            n210 = Not(x=w338) -> (.not. x?=w343:bool)
            n211 = Or(x=w355, y=w356) -> (x .or. y?=w353:bool)
            n212 = Compound Arithmetic op=OR(w367, w366, w356) -> (w333:bool)
            n213 = And(x=w344, y=w343) -> (x .and. y?=w342:bool)
            n214 = Compound Arithmetic op=OR(w369, w368, w355) -> (w335:bool)
            n215 = And(x=w353, y=w352) -> (x .and. y?=w354:bool)
            n216 = case shown="True" w342 {
              frame False {
              }
              frame True {
                n217 = property on="Iniciar / Finalizar" class="Bool (strict)"("Val(Sgnl)"=FALSE ("Value (Signaling)")) -> ()  [unwired: 2 in, 2 out]
              }
            }
            n218 = case shown="True" w354 {
              selector: w354 -> [_ w414]
              frame False {
              }
              frame True {
                n219 = property on="Iniciar / Finalizar" class="Bool (strict)"("Val(Sgnl)"=w414) -> ()  [unwired: 2 in, 2 out]
              }
            }
            n220 = property class="Bool (strict)"(reference=w339, "Value"=w333) -> ()  [unwired: 1 in, 2 out]
            n221 = property class="Bool (strict)"(reference=w340, "Value"=w335) -> ()  [unwired: 1 in, 2 out]
            n222 = case shown="False" w336 {
              tunnel: w335 -> [_ w389]
              tunnel: w333 -> [_ w388]
              tunnel: [TRUE w383] -> w316
              tunnel: w335 -> [w381 w387]
              tunnel: [w381 w386] -> w334
              tunnel: w333 -> [w380 w385]
              tunnel: [w380 w384] -> w332
              frame False {
              }
              frame True {
                n223 = Or(x=w389, y=w388) -> (x .or. y?=w390:bool)
                n224 = case shown="False" w390 {
                  tunnel: w387 -> [_ w396]
                  tunnel: [TRUE w396] -> w386
                  tunnel: w385 -> [_ w395]
                  tunnel: [FALSE w395] -> w384
                  tunnel: [FALSE TRUE] -> w383
                  frame False {
                  }
                  frame True {
                  }
                }
              }
            }
            n225 = Build Array(w334, w332, w338, w316, w303) -> (w315:bool[])
            n226 = case shown="True" w311 {
              tunnel: w316 -> [_ w377]
              tunnel: [w374 w376] -> w304
              tunnel: w315 -> [w374 _]
              tunnel: w303 -> [_ w375]
              frame False {
              }
              frame True {
                w379 = FALSE
                n227 = Build Array(w379, w379, TRUE ("element"), w377, w375) -> (w376:bool[])
              }
            }
            "Array" <- w304
            n228 = call-poly <vilib>:"DAQmx Write.vi"("task/channels in"=w365, "data"=w304, "error in"=w364) -> ("task out"=w362:refnum<k21>, "error out"=w363:errorcluster)  [unwired: 10 in, 1 out]
          }
        }
        n229 = property on="Stop" class="Bool (strict)"() -> ("Value"=w284:bool)  [unwired: 2 in, 2 out]
      }
      n230 = control-ref of="FactorsUnitatsPendents_D"() -> (w220:refnum<vi>)
      n231 = control-ref of="FactorsUnitatsPendents_F"() -> (w226:refnum<vi>)
      n232 = control-ref of="TaraF"() -> (w257:refnum<vi>)
      n233 = control-ref of="FSenseTara"() -> (w258:refnum<vi>)
      n234 = control-ref of="TablaFinal"() -> (w189:refnum<vi>)
      n235 = control-ref of="TaraD"() -> (w262:refnum<vi>)
      n236 = control-ref of="CaptadorF"() -> (w224:refnum<vi>)
      n237 = control-ref of="ParoProcessat"() -> (w207:refnum<vi>)
      n238 = while {
        shift-right: [w833] -> _
        shift-left: dbl[][] [] -> [w832]
        tunnel: w268 -> [w831]
        tunnel: w270 -> [w820]
        tunnel: w218 -> [w830]
        tunnel: w269 -> [w829]
        tunnel: w267 -> [w827]
        tunnel: [w828] -> w222
        tunnel: w266 -> [w826]
        tunnel: w265 -> [w825]
        tunnel: w263 -> [w824]
        tunnel: w264 -> [w823]
        tunnel: w260 -> [w822]
        tunnel: w259 -> [w821]
        shift-right: [w819] -> _
        shift-left: FALSE ("ControlaCaigudaSortida") -> [w818]
        tunnel: w256 -> [w817]
        tunnel: w248 -> [w816]
        tunnel: w225 -> [w815]
        tunnel: w223 -> [w814]
        tunnel: w221 -> [w813]
        tunnel: w201 -> [w811]
        tunnel: w200 -> [w810]
        tunnel: w195 -> [w808]
        tunnel: w189 -> [w807]
        stop <- w812 stop-if-true
        n239 = property on="Procesa datos" class="Bool (strict)"() -> ("Value"=w809:bool)  [unwired: 2 in, 2 out]
        n240 = property on="Ensayo activo" class="Bool (strict)"("Value"=w809) -> ()  [unwired: 2 in, 2 out]
        n241 = event shown="[0] <DadesAdquirides>: User Event" {
          selector: w827 -> [_ _ _ _]
          dyn-events: [_ _ _ _] -> w828
          timeout: _ -> [_ _ _ _]
          tunnel: w832 -> [w881 w1003 w1064 _]
          tunnel: [w880 w1002 w1063 _] -> w833
          tunnel: w809 -> [w835 w1004 _ _]
          tunnel: w831 -> [w874 _ _ _]
          tunnel: w820 -> [w875 _ _ _]
          tunnel: w830 -> [w843 _ _ _]
          tunnel: w829 -> [w876 _ _ _]
          tunnel: w826 -> [w878 _ _ _]
          tunnel: w825 -> [w855 _ _ _]
          tunnel: w824 -> [w868 _ _ _]
          tunnel: w823 -> [w877 _ _ _]
          tunnel: w822 -> [w846 _ w1060 _]
          tunnel: w821 -> [w862 _ w1061 _]
          tunnel: [w873 _ _ _] -> w819
          tunnel: w818 -> [w872 _ _ _]
          tunnel: w817 -> [w871 _ w1058 _]
          tunnel: w816 -> [w857 _ _ _]
          tunnel: w815 -> [w861 _ _ _]
          tunnel: w814 -> [_ _ _ _]
          tunnel: w813 -> [w856 _ w1059 _]
          tunnel: w811 -> [w838 _ _ _]
          tunnel: w810 -> [w837 _ _ _]
          tunnel: w808 -> [_ w1001 _ w1087]
          tunnel: w807 -> [_ _ w1057 _]
          event User Event {
            n242 = event-data() -> ("DadesAdquirides"=w853:dbl[])  [unwired: 1 in, 3 out]
            n243 = property on="Val. control sobrecarga" class="DigNum (strict)"() -> ("Value"=w859:dbl)  [unwired: 2 in, 2 out]
            n244 = Index Array(array=w853, index=0) -> (element=w836:dbl)
            n245 = call "ConverteixAD.vi"("ValorSenseTara"=w876, "ValorAdquirid"=w836, "Unitats"=w862, "Tara"=w875, "FactorsUnitatsPendents"=w874) -> ("Escala"=w860:u8, "ValorActualAbs"=w870:dbl, "ValorSenseTara"=w867:dbl)  [unwired: 4 in]
            "ValorSenseTara" <- w867
            n246 = Absolute Value(x=w867) -> (abs(x)=w840:dbl)
            n247 = property on="CaptadorD" class="Ring (strict)"() -> ("Value"=w847:u16)  [unwired: 2 in, 2 out]
            n248 = call "FormatDades.vi"("Captador"=w861, "Escala"=w860, "ValorIn"=w870, "Unidades"=w862) -> ("NDecimals"=w858:u8, "ValorOut"=w869:dbl)  [unwired: 6 in]
            n249 = property on="Sobrecarga" class="Bool (strict)"() -> ("Value"=w866:bool)  [unwired: 2 in, 2 out]
            n250 = Greater?(x=w840, y=w859) -> (0:w863:bool)
            n251 = case shown="1" w847 {
              tunnel: [1 ("index") 2 ("index")] -> w849
              tunnel: w853 -> [w895 w896]
              tunnel: [w895 w896] -> w852
              frame 0, Default {
              }
              frame 1 {
              }
            }
            n252 = Not(x=w866) -> (.not. x?=w864:bool)
            n253 = And(x=w863, y=w864) -> (x .and. y?=w865:bool)
            n254 = property on="BtMaxF" class="Bool (strict)"() -> ("Value"=w854:bool)  [unwired: 2 in, 2 out]
            n255 = Index Array(array=w852, index=w849) -> (element=w851:dbl)
            n256 = call "ConverteixAD.vi"("ValorSenseTara"=w877, "ValorAdquirid"=w851, "Unitats"=w846, "Tara"=w868, "FactorsUnitatsPendents"=w878) -> ("ValorActualAbs"=w834:dbl)  [unwired: 4 in, 2 out]
            n257 = case shown="True" w865 {
              selector: w865 -> [_ w997]
              tunnel: w863 -> [w996 _]
              frame False {
                n258 = property on="Sobrecarga" class="Bool (strict)"("Value"=w996) -> ()  [unwired: 2 in, 2 out]
              }
              frame True {
                n259 = property on="Sobrecarga" class="Bool (strict)"("Val(Sgnl)"=w997) -> ()  [unwired: 2 in, 2 out]
              }
            }
            n260 = case shown="False" w854 {
              tunnel: w843 -> [w902 w906]
              tunnel: w869 -> [w901 w903]
              tunnel: w858 -> [w900 w908]
              tunnel: w857 -> [_ w907]
              tunnel: [w899 w905] -> w842
              tunnel: [w901 w903] -> w841
              tunnel: [w898 w903] -> w839
              frame False {
                n261 = property class="DigNum (strict)"(reference=w902, "Value"=w901, "Precision"=w900) -> (error out=w899:errorcluster, "Value"=w898:sgl)  [unwired: 1 in, 1 out]
              }
              frame True {
                n262 = property class="DigNum (strict)"(reference=w907) -> (error out=w909:errorcluster, "Value"=w904:sgl)  [unwired: 1 in, 1 out]
                n263 = property class="DigNum (strict)"(reference=w906, error in=w909, "Value"=w904, "Precision"=w908) -> (error out=w905:errorcluster)  [unwired: 1 out]
              }
            }
            n264 = property on="UnidadesD" class="Ring (strict)"() -> ("Value"=w845:u16)  [unwired: 2 in, 2 out]
            n265 = case shown="2" w849 {
              tunnel: [w887 w893] -> w850
              tunnel: [w882 w890] -> w848
              tunnel: w834 -> [w886 w892]
              tunnel: w847 -> [w883 w888]
              tunnel: w845 -> [w884 w889]
              frame 1, Default {
                n266 = call "FormatDefor.vi"("UnidadesD"=w884, "ValorIn"=w886, "CaptadorD"=w883, "ResoExten"=0 ("index")) -> ("ValorOut"=w887:dbl, "NDecimals"=w882:u8)  [unwired: 6 in]
              }
              frame 2 {
                n267 = property on="ResoExten" class="Ring (strict)"() -> ("Value"=w891:i8)  [unwired: 2 in, 2 out]
                n268 = call "FormatDefor.vi"("UnidadesD"=w889, "ValorIn"=w892, "CaptadorD"=w888, "ResoExten"=w891) -> ("ValorOut"=w893:dbl, "NDecimals"=w890:u8)  [unwired: 6 in]
              }
            }
            n269 = property class="DigNum (strict)"(reference=w855, "Value"=w850, "Precision"=w848) -> (error out=w844:errorcluster)  [unwired: 1 in, 1 out]
            n270 = case shown="True" w835 {
              tunnel: w881 -> [_ w926]
              tunnel: [_ w925] -> w880
              tunnel: [FALSE ("ControlaCaigudaSortida") w921] -> w873
              tunnel: w872 -> [_ w927]
              tunnel: w871 -> [_ w928]
              tunnel: w857 -> [_ w924]
              tunnel: w855 -> [_ w923]
              tunnel: w856 -> [_ w922]
              tunnel: w844 -> [_ w918]
              tunnel: w842 -> [_ w917]
              tunnel: w841 -> [_ w916]
              tunnel: w839 -> [_ w915]
              tunnel: w838 -> [_ w914]
              tunnel: w837 -> [_ w913]
              frame False {
                n271 = property on="ParaAssaig" class="Bool (strict)"("Value"=FALSE ("ParaAssaig")) -> ()  [unwired: 2 in, 2 out]
                n272 = property on="ParoRotura" class="Bool (strict)"("Value"=FALSE ("ParoRotura")) -> ()  [unwired: 2 in, 2 out]
              }
              frame True {
                n273 = property on="Precarga" class="Bool (strict)"() -> ("Value"=w920:bool)  [unwired: 2 in, 2 out]
                n274 = case shown="True" w920 {
                  selector: w920 -> [w930 _]
                  tunnel: w916 -> [_ w931]
                  tunnel: [w929 w933] -> w919
                  frame False {
                    n275 = Not(x=w930) -> (.not. x?=w929:bool)
                  }
                  frame True {
                    n276 = property on="PrecargaOn" class="Bool (strict)"() -> ("Value"=w932:bool)  [unwired: 2 in, 2 out]
                    n277 = property on="ValorPrecarga" class="DigNum (strict)"() -> ("Value"=w937:dbl)  [unwired: 2 in, 2 out]
                    n278 = Not(x=w932) -> (.not. x?=w936:bool)
                    n279 = Greater?(x=w931, y=w937) -> (0:w934:bool)
                    n280 = And(x=w936, y=w934) -> (x .and. y?=w935:bool)
                    n281 = case shown="False" w935 {
                      selector: w935 -> [_ w940]
                      tunnel: [w938 FALSE] -> w933
                      tunnel: w932 -> [w938 _]
                      frame False {
                        n282 = property on="PrecargaOn" class="Bool (strict)"("Value"=w938) -> ()  [unwired: 2 in, 2 out]
                      }
                      frame True {
                        n283 = property on="PrecargaOn" class="Bool (strict)"("Val(Sgnl)"=w940) -> ()  [unwired: 2 in, 2 out]
                      }
                    }
                  }
                }
                n284 = case shown="True" w919 {
                  tunnel: [w941 w988] -> w921
                  tunnel: w928 -> [_ w987]
                  tunnel: w927 -> [w941 w986]
                  tunnel: w926 -> [w942 w985]
                  tunnel: [w942 w984] -> w925
                  tunnel: w924 -> [_ w983]
                  tunnel: w923 -> [_ w982]
                  tunnel: w922 -> [_ w981]
                  tunnel: w918 -> [_ w967]
                  tunnel: w917 -> [_ _]
                  tunnel: w915 -> [_ w958]
                  tunnel: w914 -> [_ w963]
                  tunnel: w913 -> [_ w950]
                  frame False {
                  }
                  frame True {
                    w977 = 0
                    n285 = property class="DigNum (strict)"(reference=w981) -> ("Value"=w968:sgl)  [unwired: 1 in, 2 out]
                    n286 = property class="DigNum (strict)"(reference=w963) -> (reference out=w960:refnum<vi>, "Value"=w962:dbl)  [unwired: 1 in, 1 out]
                    n287 = property class="DigNum (strict)"(reference=w983) -> (reference out=w971:refnum<vi>, "Value"=w972:sgl)  [unwired: 1 in, 1 out]
                    n288 = property class="DigNum (strict)"(reference=w950) -> ("Value"=w957:sgl)  [unwired: 1 in, 2 out]
                    n289 = property class="DigNum (strict)"(reference=w987) -> ("Value"=w974:sgl)  [unwired: 1 in, 2 out]
                    n290 = property on="ActivaParoDefor" class="Bool (strict)"() -> ("Value"=w964:bool)  [unwired: 2 in, 2 out]
                    n291 = Not Equal To 0?(x=w968) -> (x != 0?=w965:bool)
                    n292 = property on="Fent_Rep" class="Bool (strict)"() -> ("Value"=w944:bool)  [unwired: 2 in, 2 out]
                    n293 = property class="DigNum (strict)"(reference=w982, error in=w967) -> ("Value"=w969:sgl)  [unwired: 2 out]
                    n294 = And(x=w964, y=w965) -> (x .and. y?=w945:bool)
                    n295 = Increment(x=w962) -> (x+1=w961:dbl)
                    n296 = Not(x=w944) -> (.not. x?=w943:bool)
                    n297 = property on="ParoDeforFet" class="Bool (strict)"() -> ("Value"=w948:bool)  [unwired: 2 in, 2 out]
                    n298 = property on="ActivaParoCarga" class="Bool (strict)"() -> ("Value"=w959:bool)  [unwired: 2 in, 2 out]
                    n299 = property on="ParoCargaFet" class="Bool (strict)"() -> ("Value"=w954:bool)  [unwired: 2 in, 2 out]
                    n300 = Greater Or Equal?(x=w958, y=w957) -> (x >= y?=w956:bool)
                    n301 = property class="DigNum (strict)"(reference=w960, "Value"=w961) -> ()  [unwired: 1 in, 2 out]
                    n302 = call "ControlFiAssaig.vi"("Actiu"=w943, "PercentatgeCaiguda"=w974, "ControlaCaigudaEntrada"=w986, "ValorActual"=w958, "ValorMaxim"=w972) -> ("ControlaCaigudaSortida"=w988:bool, "ParoRotura"=w966:bool, "NouMaxim"=w970:dbl)  [unwired: 4 in]
                    n303 = Not(x=w948) -> (.not. x?=w946:bool)
                    n304 = Not(x=w954) -> (.not. x?=w952:bool)
                    n305 = And(x=w959, y=w956) -> (x .and. y?=w953:bool)
                    n306 = And(x=w945, y=w946) -> (x .and. y?=w947:bool)
                    n307 = And(x=w953, y=w952) -> (x .and. y?=w951:bool)
                    n308 = property class="DigNum (strict)"(reference=w971, "Value"=w970) -> ()  [unwired: 1 in, 2 out]
                    n309 = case shown="True" w947 {
                      tunnel: w968 -> [_ w993]
                      tunnel: w969 -> [_ w992]
                      frame False {
                      }
                      frame True {
                        n310 = Greater?(x=w992, y=w993) -> (0:w991:bool)
                        n311 = case shown="True" w991 {
                          selector: w991 -> [_ w994]
                          frame False {
                          }
                          frame True {
                            n312 = property on="ParoDefor" class="Bool (strict)"("Val(Sgnl)"=w994) -> ()  [unwired: 2 in, 2 out]
                          }
                        }
                      }
                    }
                    n313 = Array Size(array=w985) -> (size(s)=w978:i32[])
                    n314 = case shown="True" w951 {
                      selector: w951 -> [_ w990]
                      frame False {
                      }
                      frame True {
                        n315 = property on="ParoCarga" class="Bool (strict)"("Val(Sgnl)"=w990) -> ()  [unwired: 2 in, 2 out]
                      }
                    }
                    n316 = property on="ActivaParoRotura" class="Bool (strict)"() -> ("Value"=w949:bool)  [unwired: 2 in, 2 out]
                    n317 = Index Array(array=w978, index=w977) -> (element=w976:i32)
                    n318 = Equal?(x=w976, y=w977) -> (x = y?=w975:bool)
                    n319 = And(x=w949, y=w966) -> (x .and. y?=w955:bool)
                    n320 = call "Build XY Graph"("Reset"=w975, "Y Input"=w958, "X Input"=w969) -> ("XY Graph"=→"?":cluster{"Y":dbl[], "Y":dbl[]}[])  [unwired: 7 in, 1 out]
                    n321 = Merge Signals(w969, w958) -> (w979:dynamicdata)
                    n322 = case shown="True" w955 {
                      selector: w955 -> [_ w995]
                      frame False {
                      }
                      frame True {
                        n323 = property on="ParoRotura" class="Bool (strict)"("Val(Sgnl)"=w995) -> ()  [unwired: 2 in, 2 out]
                      }
                    }
                    n324 = property on="First time" class="Bool (strict)"("Value"=TRUE) -> ()  [unwired: 2 in, 2 out]
                    n325 = call "Convert from Dynamic Data"("Dynamic Data Type"=w979) -> ("Array"=w973:dbl[])  [unwired: 3 in]
                    n326 = Build Array (concatenate)(w985, w973) -> (w984:dbl[][])
                    "Tabla" <- w984
                  }
                }
              }
            }
          }
          event "Salir": Value Change {
            n327 = event-data() -> ()  [unwired: 1 in, 6 out]
            n328 = property on="rings" class="Arr (strict)"() -> ("Value"=w1000:refnum<vi>[])  [unwired: 2 in, 2 out]
            n329 = property on="Caselles" class="Arr (strict)"() -> ("Value"=w999:refnum<vi>[])  [unwired: 2 in, 2 out]
            n330 = property on="Booleans" class="Arr (strict)"() -> ("Value"=w998:refnum<vi>[])  [unwired: 2 in, 2 out]
            n331 = case shown="True" w1004 {
              selector: w1004 -> [_ w1032]
              tunnel: w1003 -> [_ w1034]
              tunnel: [_ w1034] -> w1002
              tunnel: w1001 -> [_ w1031]
              tunnel: w1000 -> [w1007 w1028]
              tunnel: w999 -> [w1006 w1027]
              tunnel: w998 -> [w1005 w1026]
              frame False {
                n332 = flat-sequence {
                  tunnel: w1007 -> [w1010]
                  tunnel: w1006 -> [w1009]
                  tunnel: w1005 -> [w1008]
                  frame #0 {
                    n333 = call "GuardaValorsPantalla.vi"("Rings"=w1010, "Caselles"=w1009, "Booleans"=w1008) -> ()  [unwired: 7 in, 1 out]
                  }
                  frame #1 {
                    n334 = call <vilib>:"DAQmx Stop Task.vi"("task/channels in"=refnum<k21> "USBAnalogIn") -> ("task out"=w1022:refnum<k21>, "error out"=w1021:errorcluster)  [unwired: 13 in]
                    n335 = call <vilib>:"DAQmx Stop Task.vi"("task/channels in"=refnum<k21> "USBAnalogOut") -> ("task out"=w1017:refnum<k21>, "error out"=w1019:errorcluster)  [unwired: 13 in]
                    n336 = call <vilib>:"DAQmx Stop Task.vi"("task/channels in"=refnum<k21> "USBDigitalIn") -> ("task out"=w1015:refnum<k21>, "error out"=w1016:errorcluster)  [unwired: 13 in]
                    n337 = call <vilib>:"DAQmx Stop Task.vi"("task/channels in"=refnum<k21> "USBEncoder") -> ("task out"=w1013:refnum<k21>)  [unwired: 13 in, 1 out]
                    n338 = call <vilib>:"DAQmx Stop Task.vi"("task/channels in"=refnum<k21> "USBDigitalOut") -> ("task out"=w1024:refnum<k21>, "error out"=w1023:errorcluster)  [unwired: 13 in]
                    n339 = call <vilib>:"DAQmx Clear Task.vi"("task in"=w1022, "error in"=w1021) -> ()  [unwired: 13 in, 1 out]
                    n340 = call <vilib>:"DAQmx Clear Task.vi"("task in"=w1017, "error in"=w1019) -> ()  [unwired: 13 in, 1 out]
                    n341 = call <vilib>:"DAQmx Clear Task.vi"("task in"=w1015, "error in"=w1016) -> ()  [unwired: 13 in, 1 out]
                    n342 = call <vilib>:"DAQmx Clear Task.vi"("task in"=w1024, "error in"=w1023) -> ()  [unwired: 13 in, 1 out]
                    n343 = call <vilib>:"DAQmx Clear Task.vi"("task in"=w1013) -> ()  [unwired: 14 in, 1 out]
                  }
                  frame #2 {
                    n344 = Quit LabVIEW(quit? (T)=TRUE) -> ()
                  }
                }
              }
              frame True {
                # "Mensaje de cancelar o no el ensayo activo"
                n345 = Index Array(array=w1031, index=2) -> (element=w1029:string)
                n346 = call "Display Message to User2"("Enable"=w1032, "Message"=w1029) -> ("OK"=w1033:bool)  [unwired: 8 in, 1 out]
                n347 = case shown="True" w1033 {
                  tunnel: w1028 -> [_ w1038]
                  tunnel: w1027 -> [_ w1037]
                  tunnel: w1026 -> [_ w1036]
                  frame False {
                    n348 = property on="Salir" class="Bool (strict)"("Value"=FALSE ("Salir")) -> ()  [unwired: 2 in, 2 out]
                  }
                  frame True {
                    n349 = flat-sequence {
                      tunnel: w1038 -> [w1041]
                      tunnel: w1037 -> [w1040]
                      tunnel: w1036 -> [w1039]
                      frame #0 {
                        n350 = call "GuardaValorsPantalla.vi"("Rings"=w1041, "Caselles"=w1040, "Booleans"=w1039) -> ()  [unwired: 7 in, 1 out]
                      }
                      frame #1 {
                        n351 = call <vilib>:"DAQmx Stop Task.vi"("task/channels in"=refnum<k21> "USBAnalogIn") -> ("task out"=w1053:refnum<k21>, "error out"=w1052:errorcluster)  [unwired: 13 in]
                        n352 = call <vilib>:"DAQmx Stop Task.vi"("task/channels in"=refnum<k21> "USBAnalogOut") -> ("task out"=w1048:refnum<k21>, "error out"=w1050:errorcluster)  [unwired: 13 in]
                        n353 = call <vilib>:"DAQmx Stop Task.vi"("task/channels in"=refnum<k21> "USBDigitalIn") -> ("task out"=w1046:refnum<k21>, "error out"=w1047:errorcluster)  [unwired: 13 in]
                        n354 = call <vilib>:"DAQmx Stop Task.vi"("task/channels in"=refnum<k21> "USBEncoder") -> ("task out"=w1044:refnum<k21>)  [unwired: 13 in, 1 out]
                        n355 = call <vilib>:"DAQmx Stop Task.vi"("task/channels in"=refnum<k21> "USBDigitalOut") -> ("task out"=w1055:refnum<k21>, "error out"=w1054:errorcluster)  [unwired: 13 in]
                        n356 = call <vilib>:"DAQmx Clear Task.vi"("task in"=w1053, "error in"=w1052) -> ()  [unwired: 13 in, 1 out]
                        n357 = call <vilib>:"DAQmx Clear Task.vi"("task in"=w1048, "error in"=w1050) -> ()  [unwired: 13 in, 1 out]
                        n358 = call <vilib>:"DAQmx Clear Task.vi"("task in"=w1046, "error in"=w1047) -> ()  [unwired: 13 in, 1 out]
                        n359 = call <vilib>:"DAQmx Clear Task.vi"("task in"=w1055, "error in"=w1054) -> ()  [unwired: 13 in, 1 out]
                        n360 = call <vilib>:"DAQmx Clear Task.vi"("task in"=w1044) -> ()  [unwired: 14 in, 1 out]
                      }
                      frame #2 {
                        n361 = Quit LabVIEW(quit? (T)=TRUE) -> ()
                      }
                    }
                  }
                }
              }
            }
          }
          event "Guardar": Value Change {
            n362 = event-data() -> ("NewVal"=w1062:bool)  [unwired: 1 in, 5 out]
            n363 = case shown="True" w1062 {
              tunnel: w1064 -> [w1065 w1084]
              tunnel: [w1065 w1083] -> w1063
              tunnel: w1061 -> [_ w1081]
              tunnel: w1060 -> [_ w1082]
              tunnel: w1059 -> [_ w1073]
              tunnel: w1058 -> [_ w1071]
              tunnel: [_ w1067] -> _
              tunnel: w1057 -> [_ w1067]
              frame False {
              }
              frame True {
                w1078 = ""
                n364 = property on="ActivaParoRotura" class="Bool (strict)"() -> ("Value"=w1077:bool)  [unwired: 2 in, 2 out]
                n365 = property on="Velocidad Ensayo" class="DigNum (strict)"() -> ("Value"=w1080:sgl)  [unwired: 2 in, 2 out]
                n366 = property on="Precarga" class="Bool (strict)"() -> ("Value"=w1076:bool)  [unwired: 2 in, 2 out]
                n367 = property on="ActivaParoDefor" class="Bool (strict)"() -> ("Value"=w1079:bool)  [unwired: 2 in, 2 out]
                n368 = property class="DigNum (strict)"(reference=w1073) -> ("Value"=w1072:sgl)  [unwired: 1 in, 2 out]
                n369 = property class="Arr (strict)"(reference=w1067) -> ("Value"=w1066:dbl[][])  [unwired: 1 in, 2 out]
                n370 = property class="DigNum (strict)"(reference=w1071) -> ("Value"=w1070:sgl)  [unwired: 1 in, 2 out]
                n371 = property on="ValorPrecarga" class="DigNum (strict)"() -> ("Value"=w1069:dbl)  [unwired: 2 in, 2 out]
                n372 = property on="ArraiMostresxProva" class="Arr (strict)"() -> ("Value"=w1068:dbl[])  [unwired: 2 in, 2 out]
                n373 = property on="Nº Tests" class="DigNum (strict)"() -> ("Value"=w1074:u8)  [unwired: 2 in, 2 out]
                n374 = call "CreaInformeExcel.vi"("UnidadesF"=w1081, "ValorParoDesplazamiento"=w1072, "TipusAssaig"=w1078, "ActivaParoDefor"=w1079, 4:w1080, "ArraiMostresxProva"=w1068, "Nom Assaig"=w1078, "Precarga"=w1076, "NºTests"=w1074, "ValorPrecarga"=w1069, "UnidadesD"=w1082, "ActivaParoRotura"=w1077, "TablaFinal"=w1066, "ValorParoRotura"=w1070) -> ("status"=w1075:bool)  [unwired: 5 in]
                n375 = case shown="True" w1075 {
                  tunnel: w1084 -> [w1085 _]
                  tunnel: [w1085 dbl[][] []] -> w1083
                  frame False {
                  }
                  frame True {
                  }
                }
              }
            }
          }
          event "BtEliminarUltima": Value Change {
            n376 = event-data() -> ("NewVal"=w1088:bool)  [unwired: 1 in, 5 out]
            n377 = case shown="True" w1088 {
              tunnel: w1087 -> [_ w1089]
              frame False {
              }
              frame True {
                n378 = property on="Nº Tests" class="DigNum (strict)"() -> ("Value"=w1090:u8)  [unwired: 2 in, 2 out]
                n379 = Greater Than 0?(x=w1090) -> (x > 0?=w1091:bool)
                n380 = case shown="True" w1091 {
                  tunnel: w1090 -> [_ w1099]
                  tunnel: w1089 -> [w1094 w1097]
                  frame False {
                    n381 = Index Array(array=w1094, index=4) -> (element=w1092:string)
                    n382 = call "Display Message to User3"("Message"=w1092) -> ()  [unwired: 9 in, 2 out]
                  }
                  frame True {
                    n383 = Index Array(array=w1097, index=3) -> (element=w1095:string)
                    n384 = call "Display Message to User6"("Message"=w1095) -> ("OK"=w1098:bool)  [unwired: 9 in, 1 out]
                    n385 = case shown="True" w1098 {
                      tunnel: w1099 -> [_ w1107]
                      frame False {
                      }
                      frame True {
                        w1110 = u8 2 ("y")
                        n386 = Subtract(x=w1107, y=1.0) -> (x-y=w1109:dbl)
                        n387 = Multiply(x=w1107, y=w1110) -> (x*y=w1111:u8)
                        n388 = property on="TablaFinal" class="Arr (strict)"() -> ("Value"=w1103:dbl[][])  [unwired: 2 in, 2 out]
                        n389 = property on="Nº Tests" class="DigNum (strict)"("Value"=w1109) -> ()  [unwired: 2 in, 2 out]
                        n390 = Subtract(x=w1111, y=w1110) -> (x-y=w1101:u8)
                        n391 = property on="Columna" class="DigNum (strict)"("Value"=w1101) -> ()  [unwired: 2 in, 2 out]
                        n392 = Initialize Array(0.0 ("element"), 3600 ("dimension size"), 2 ("dimension size")) -> ()  [unwired: 1 out]
                        n393 = Delete From Array(array=w1103, length=3600, index (col)=w1101) -> (array with subset deleted=w1102:dbl[][])  [unwired: 1 in, 1 out]
                        n394 = property on="TablaFinal" class="Arr (strict)"("Value"=w1102) -> ()  [unwired: 2 in, 2 out]
                      }
                    }
                  }
                }
              }
            }
          }
        }
        n395 = property on="Stop" class="Bool (strict)"() -> ("Value"=w812:bool)  [unwired: 2 in, 2 out]
      }
      n396 = control-ref of="NMostres"() -> (w192:refnum<vi>)
      n397 = control-ref of="Tabla"() -> (w190:refnum<vi>)
      n398 = control-ref of="ParoCargaFet"() -> (w194:refnum<vi>)
      n399 = control-ref of="TablaFinal"() -> (w191:refnum<vi>)
      n400 = while {
        tunnel: w261 -> [w518]
        tunnel: w262 -> [w517]
        tunnel: w258 -> [w516]
        tunnel: w257 -> [w515]
        tunnel: w226 -> [w514]
        tunnel: w224 -> [w513]
        tunnel: w220 -> [w512]
        tunnel: w207 -> [w511]
        tunnel: w195 -> [w510]
        tunnel: w194 -> [w509]
        tunnel: w192 -> [w508]
        tunnel: w191 -> [w507]
        tunnel: w190 -> [w506]
        stop <- w519 stop-if-true
        n401 = event shown="[11] \"BtTaraD\": Value Change" {
          selector: _ -> [_ _ _ _ _ _ _ _ _ _ _ _ _ _]
          dyn-events: _ -> [_ _ _ _ _ _ _ _ _ _ _ _ _ _]
          timeout: _ -> [_ _ _ _ _ _ _ _ _ _ _ _ _ _]
          tunnel: w518 -> [_ _ _ _ _ _ _ _ _ _ _ w794 _ w801]
          tunnel: w517 -> [_ _ _ _ _ _ w722 _ _ _ _ w791 _ w800]
          tunnel: w516 -> [_ _ _ _ _ _ _ _ _ _ _ _ w797 w799]
          tunnel: w515 -> [_ _ _ _ _ w706 _ _ _ _ _ _ w796 w798]
          tunnel: [_ _ _ _ _ _ _ w729 _ w770 _ _ _ _] -> _
          tunnel: w514 -> [_ _ _ _ _ _ _ w729 _ w770 _ _ _ _]
          tunnel: w513 -> [_ _ _ _ _ w707 _ w725 _ _ _ _ _ _]
          tunnel: w512 -> [_ _ _ _ _ _ _ _ _ w769 _ _ _ _]
          tunnel: [_ _ _ _ _ _ _ _ _ _ _ w794 _ _] -> _
          tunnel: w511 -> [_ _ _ _ _ _ _ _ _ _ w776 _ _ _]
          tunnel: w510 -> [w523 w572 w588 w658 _ _ _ _ _ _ _ _ _ _]
          tunnel: w509 -> [_ _ w586 _ _ _ _ _ _ _ _ _ _ _]
          tunnel: w508 -> [w522 _ _ _ _ _ _ _ _ _ _ _ _ _]
          tunnel: w507 -> [w521 w571 _ _ _ _ _ _ _ _ _ _ _ _]
          tunnel: w506 -> [w520 _ _ _ _ _ _ _ _ _ _ _ _ _]
          event "Iniciar / Finalizar": Value Change {
            n402 = event-data() -> ()  [unwired: 1 in, 5 out]
            n403 = property on="Iniciar / Finalizar" class="Bool (strict)"() -> ("Value"=w524:bool)  [unwired: 2 in, 2 out]
            n404 = case shown="False" w524 {
              tunnel: w523 -> [_ w567]
              tunnel: w522 -> [w529 _]
              tunnel: w521 -> [w526 _]
              tunnel: w520 -> [w525 _]
              frame False {
                n405 = flat-sequence {
                  tunnel: w529 -> [w534]
                  tunnel: [w532] -> w527
                  tunnel: w526 -> [w531]
                  tunnel: w525 -> [w530]
                  tunnel: [w557] -> w528
                  tunnel: w527 -> [w557]
                  tunnel: w528 -> [w560]
                  frame #0 {
                    w535 = FALSE ("ParoCarga")
                    n406 = property on="ParoCarga" class="Bool (strict)"("Value"=w535) -> ()  [unwired: 2 in, 2 out]
                    n407 = property on="ParoCargaFet" class="Bool (strict)"("Value"=w535) -> ()  [unwired: 2 in, 2 out]
                    n408 = property on="ParoDefor" class="Bool (strict)"("Value"=w535) -> ()  [unwired: 2 in, 2 out]
                    n409 = property on="ParoDeforFet" class="Bool (strict)"("Value"=w535) -> ()  [unwired: 2 in, 2 out]
                    n410 = property on="First time" class="Bool (strict)"() -> ("Value"=w533:bool)  [unwired: 2 in, 2 out]
                    n411 = property on="Procesa datos" class="Bool (strict)"("Value"=FALSE) -> ()  [unwired: 2 in, 2 out]
                    n412 = property on="ParaAssaig" class="Bool (strict)"("Value"=TRUE ("ParaAssaig")) -> ()  [unwired: 2 in, 2 out]
                    n413 = case shown="True" w533 {
                      tunnel: [_ w546] -> _
                      tunnel: w534 -> [_ w546]
                      tunnel: [_ w544] -> w532
                      tunnel: w531 -> [_ w543]
                      tunnel: w530 -> [_ w539]
                      frame False {
                      }
                      frame True {
                        n414 = property class="DigNum (strict)"(reference=w546) -> (reference out=w544:refnum<vi>, "Value"=w545:dbl)  [unwired: 1 in, 1 out]
                        n415 = property on="Nº Tests" class="DigNum (strict)"() -> ("Value"=w551:u8)  [unwired: 2 in, 2 out]
                        n416 = Increment(x=w551) -> (x+1=w553:u8)
                        n417 = property on="Nº Tests" class="DigNum (strict)"("Value"=w553) -> ()  [unwired: 2 in, 2 out]
                        n418 = property on="ArraiMostresxProva" class="Arr (strict)"() -> ("Value"=w552:dbl[])  [unwired: 2 in, 2 out]
                        n419 = Insert Into Array(array=w552, index=w551, new element=w545) -> (w550:dbl[])
                        n420 = property on="ArraiMostresxProva" class="Arr (strict)"("Value"=w550) -> ()  [unwired: 2 in, 2 out]
                        n421 = property on="StringsEstatMáquina" class="Arr (strict)"() -> ("Value"=w549:string[])  [unwired: 2 in, 2 out]
                        n422 = property on="CodiAturada" class="DigNum (strict)"() -> ("Value"=w547:u32)  [unwired: 2 in, 2 out]
                        n423 = property class="Arr (strict)"(reference=w539) -> ("Value"=w538:dbl[][])  [unwired: 1 in, 2 out]
                        n424 = property class="Arr (strict)"(reference=w543) -> (reference out=w541:refnum<vi>, "Value"=w542:dbl[][])  [unwired: 1 in, 1 out]
                        n425 = Index Array(array=w549, index=w547) -> (element=w548:string)
                        n426 = property on="Columna" class="DigNum (strict)"() -> ("Value"=w554:i32)  [unwired: 2 in, 2 out]
                        n427 = property on="Estado ensayo:" class="Str"("Value"=w548) -> ()  [unwired: 2 in, 2 out]
                        n428 = Insert Into Array(array=w542, index (col)=w554, new element=w538) -> (w540:dbl[][])  [unwired: 1 in]
                        n429 = property class="Arr (strict)"(reference=w541, "Value"=w540) -> ()  [unwired: 1 in, 2 out]
                        n430 = Add(x=w554, y=2) -> (x+y=w555:i32)
                        n431 = property on="Columna" class="DigNum (strict)"("Value"=w555) -> ()  [unwired: 2 in, 2 out]
                      }
                    }
                  }
                  frame #1 {
                    n432 = Wait (ms)(milliseconds to wait=u32 200) -> ()  [unwired: 1 out]
                  }
                  frame #2 {
                    n433 = property class="DigNum (strict)"(reference=w560, "Value"=0.0 ("NMostres")) -> ()  [unwired: 1 in, 2 out]
                    n434 = property on="Tabla" class="Arr (strict)"("Value"=dbl[][] [] ("Tabla")) -> ()  [unwired: 2 in, 2 out]
                    n435 = property on="Rep. Fetes" class="DigNum (strict)"("Value"=u8 0 ("Rep. Fetes")) -> ()  [unwired: 2 in, 2 out]
                    n436 = property on="PrecargaOn" class="Bool (strict)"("Value"=FALSE ("PrecargaOn")) -> ()  [unwired: 2 in, 2 out]
                    n437 = property on="First time" class="Bool (strict)"("Value"=FALSE) -> ()  [unwired: 2 in, 2 out]
                  }
                }
              }
              frame True {
                n438 = Index Array(array=w567, index=18) -> (element=w566:string)
                n439 = property on="Estado ensayo:" class="Str"("Value"=w566) -> ()  [unwired: 2 in, 2 out]
                n440 = property on="Maxim" class="DigNum (strict)"("Value"=0.0 ("Maxim")) -> (error out=w568:errorcluster)  [unwired: 2 in, 1 out]
                n441 = property on="Procesa datos" class="Bool (strict)"(error in=w568, "Value"=TRUE) -> ()  [unwired: 1 in, 2 out]
              }
            }
          }
          event "Ensayonuevo": Value Change {
            n442 = event-data() -> ("NewVal"=w573:bool)  [unwired: 1 in, 5 out]
            n443 = case shown="True" w573 {
              tunnel: w572 -> [_ w577]
              tunnel: [_ w574] -> _
              tunnel: w571 -> [_ w574]
              frame False {
              }
              frame True {
                n444 = Index Array(array=w577, index=0) -> (element=w575:string)
                n445 = call "Display Message to User"("Message"=w575) -> ("OK"=w578:bool)  [unwired: 9 in, 1 out]
                n446 = case shown="True" w578 {
                  tunnel: w574 -> [_ w580]
                  frame False {
                  }
                  frame True {
                    n447 = property on="Columna" class="DigNum (strict)"("Value"=0 ("Columna")) -> ()  [unwired: 2 in, 2 out]
                    n448 = Initialize Array(0.0 ("element"), 3600 ("dimension size"), 2 ("dimension size")) -> (w579:dbl[][])
                    n449 = property on="Nº Tests" class="DigNum (strict)"("Value"=u8 0 ("Nº Tests")) -> ()  [unwired: 2 in, 2 out]
                    n450 = property class="Arr (strict)"(reference=w580, "Value"=w579) -> ()  [unwired: 1 in, 2 out]
                  }
                }
              }
            }
          }
          event "ParoCarga": Value Change {
            n451 = event-data() -> ("NewVal"=w587:bool)  [unwired: 1 in, 5 out]
            n452 = case shown="True" w587 {
              tunnel: w588 -> [_ w592]
              tunnel: w586 -> [_ w591]
              frame False {
              }
              frame True {
                n453 = property class="Bool (strict)"(reference=w591) -> (reference out=w589:refnum<vi>, "Value"=w590:bool)  [unwired: 1 in, 1 out]
                n454 = case shown="False" w590 {
                  tunnel: w592 -> [w593 _]
                  tunnel: w589 -> [w596 _]
                  frame False {
                    n455 = property on="FinalEnsayo" class="Bool (strict)"() -> (error out=w595:errorcluster, "Value"=w604:bool)  [unwired: 2 in, 1 out]
                    n456 = property class="Bool (strict)"(reference=w596, error in=w595, "Value"=TRUE ("ParoCargaFet")) -> (reference out=w594:refnum<vi>, error out=w598:errorcluster)
                    n457 = Index Array(array=w593, index=1) -> (element=w600:string)
                    n458 = case shown="False" w604 {
                      tunnel: [w616 FALSE ("SI")] -> w605
                      tunnel: [w611 w650] -> w602
                      tunnel: w600 -> [w615 _]
                      tunnel: w598 -> [w610 w650]
                      tunnel: w594 -> [w609 _]
                      tunnel: w593 -> [w608 _]
                      frame False {
                        n459 = property on="Rep. A Fer" class="DigNum (strict)"() -> ("Value"=w614:sgl)  [unwired: 2 in, 2 out]
                        n460 = Index Array(array=w608, index=5) -> (element=w606:string)
                        n461 = Greater?(x=w614, y=u8 0) -> (0:w612:bool)
                        n462 = case shown="True" w612 {
                          tunnel: [w632 w648] -> w616
                          tunnel: w615 -> [w622 w647]
                          tunnel: w614 -> [w631 _]
                          tunnel: w610 -> [w628 w646]
                          tunnel: [w627 w646] -> w611
                          tunnel: w609 -> [w626 _]
                          tunnel: w606 -> [w619 _]
                          frame True {
                            n463 = property on="Rep. Fetes" class="DigNum (strict)"() -> ("Value"=w629:u8)  [unwired: 2 in, 2 out]
                            n464 = Increment(x=w629) -> (x+1=w621:u8)
                            n465 = property on="Fent_Rep" class="Bool (strict)"("Value"=TRUE ("Fent_Rep")) -> ()  [unwired: 2 in, 2 out]
                            n466 = Greater Or Equal?(x=w621, y=w631) -> (x >= y?=w630:bool)
                            n467 = Format Into String(w621) -> (resulting string=w618:string)  [unwired: 3 in, 1 out]
                            n468 = Concatenate Strings(w619, w618) -> (w620:string)
                            n469 = Concatenate Strings(w620, "\r", w622) -> (w617:string)
                            n470 = case shown="True" w630 {
                              tunnel: [w638 w645] -> w632
                              tunnel: w621 -> [w636 w640]
                              tunnel: w628 -> [w637 _]
                              tunnel: [w637 w644] -> w627
                              tunnel: w626 -> [_ w643]
                              tunnel: [w636 w640] -> w625
                              tunnel: w617 -> [w633 w639]
                              frame True {
                                n471 = call "Display Message to User5"("Message"=w633) -> ("error out"=w634:errorcluster, "SI"=w638:bool)  [unwired: 9 in]
                                n472 = property on="Fent_Rep" class="Bool (strict)"(error in=w634, "Value"=FALSE ("Fent_Rep")) -> ()  [unwired: 1 in, 2 out]
                              }
                              frame False {
                                n473 = call "Display Message to User8"("Message"=w639) -> ("error out"=w641:errorcluster, "SI"=w645:bool)  [unwired: 9 in]
                                n474 = property class="Bool (strict)"(reference=w643, error in=w641, "Value"=FALSE) -> (error out=w644:errorcluster)  [unwired: 1 out]
                              }
                            }
                            n475 = property on="Rep. Fetes" class="DigNum (strict)"("Value"=w625) -> ()  [unwired: 2 in, 2 out]
                          }
                          frame False {
                            n476 = call "Display Message to User7"("Message"=w647) -> ("SI"=w648:bool)  [unwired: 9 in, 1 out]
                          }
                        }
                      }
                      frame True {
                      }
                    }
                    n477 = case shown="False" w605 {
                      tunnel: w602 -> [w653 w657]
                      tunnel: [w653 w657] -> w599
                      frame False {
                        n478 = property on="Procesa datos" class="Bool (strict)"("Value"=FALSE ("Procesa datos")) -> (error out=w655:errorcluster)  [unwired: 2 in, 1 out]
                        n479 = property on="Iniciar / Finalizar" class="Bool (strict)"(error in=w655, "Val(Sgnl)"=FALSE ("Value (Signaling)")) -> (error out=w651:errorcluster)  [unwired: 1 in, 1 out]
                        n480 = property on="Rep. Fetes" class="DigNum (strict)"(error in=w651, "Value"=u8 0 ("Rep. Fetes")) -> ()  [unwired: 1 in, 2 out]
                      }
                      frame True {
                      }
                    }
                    n481 = property on="ParoCarga" class="Bool (strict)"(error in=w599, "Value"=FALSE ("ParoCarga")) -> ()  [unwired: 1 in, 2 out]
                  }
                  frame True {
                  }
                }
              }
            }
          }
          event "ParoDefor": Value Change {
            n482 = event-data() -> ("NewVal"=w659:bool)  [unwired: 1 in, 5 out]
            n483 = case shown="True" w659 {
              tunnel: w658 -> [_ w660]
              frame False {
              }
              frame True {
                n484 = property on="ParoDeforFet" class="Bool (strict)"() -> (error out=w662:errorcluster, "Value"=w661:bool)  [unwired: 2 in, 1 out]
                n485 = case shown="False" w661 {
                  tunnel: w662 -> [w672 _]
                  tunnel: w660 -> [w665 _]
                  frame False {
                    n486 = property on="FinalEnsayo" class="Bool (strict)"(error in=w672) -> (error out=w670:errorcluster, "Value"=w673:bool)  [unwired: 1 in, 1 out]
                    n487 = property on="ParoDeforFet" class="Bool (strict)"(error in=w670, "Value"=TRUE ("ParoCargaFet")) -> (error out=w669:errorcluster)  [unwired: 1 in, 1 out]
                    n488 = Index Array(array=w665, index=1) -> (element=w663:string)
                    n489 = case shown="False" w673 {
                      tunnel: [w677 FALSE ("SI")] -> w674
                      tunnel: w669 -> [w676 w678]
                      tunnel: [w676 w678] -> w671
                      tunnel: w663 -> [w675 _]
                      frame False {
                        n490 = call "Display Message to User4"("Message"=w675) -> ("SI"=w677:bool)  [unwired: 9 in, 1 out]
                      }
                      frame True {
                      }
                    }
                    n491 = case shown="False" w674 {
                      tunnel: w671 -> [w680 w684]
                      tunnel: [w680 w684] -> w666
                      frame False {
                        n492 = property on="Procesa datos" class="Bool (strict)"("Value"=FALSE ("Procesa datos")) -> (error out=w682:errorcluster)  [unwired: 2 in, 1 out]
                        n493 = property on="Iniciar / Finalizar" class="Bool (strict)"(error in=w682, "Val(Sgnl)"=FALSE ("Value (Signaling)")) -> ()  [unwired: 1 in, 2 out]
                      }
                      frame True {
                      }
                    }
                    n494 = property on="ParoDefor" class="Bool (strict)"(error in=w666, "Value"=FALSE ("ParoCarga")) -> ()  [unwired: 1 in, 2 out]
                  }
                  frame True {
                  }
                }
              }
            }
          }
          event "ParoRotura": Value Change {
            n495 = event-data() -> ("NewVal"=w685:bool)  [unwired: 1 in, 5 out]
            n496 = case shown="True" w685 {
              frame False {
              }
              frame True {
                n497 = property on="Procesa datos" class="Bool (strict)"("Value"=FALSE ("Procesa datos")) -> (error out=w687:errorcluster)  [unwired: 2 in, 1 out]
                n498 = property on="Iniciar / Finalizar" class="Bool (strict)"(error in=w687, "Val(Sgnl)"=FALSE ("Value (Signaling)")) -> ()  [unwired: 1 in, 2 out]
              }
            }
          }
          event "UnidadesF": Value Change {
            n499 = event-data() -> ("NewVal"=w694:u16)  [unwired: 1 in, 5 out]
            n500 = property class="Ring (strict)"(reference=w707) -> ("Strings []"=w692:string[], "RingText.Text"=w691:string)  [unwired: 1 in, 2 out]
            n501 = Search 1D Array(1D array=w692, element=w691) -> (index of element=w693:i32)  [unwired: 1 in]
            n502 = property on="ConversioUnitatsF" class="Arr (strict)"() -> ("Value"=w708:dbl[])  [unwired: 2 in, 2 out]
            n503 = property class="DigNum (strict)"(reference=w706, "Value"=sgl 0.0) -> ()  [unwired: 1 in, 2 out]
            n504 = case shown="0, Default" w693 {
              tunnel: [w710 w711] -> w704
              frame 0, Default {
                n505 = property on="ValorSobrecargaC1" class="DigNum (strict)"() -> ("Value"=w710:dbl)  [unwired: 2 in, 2 out]
              }
              frame 1 {
                n506 = property on="ValorSobrecargaC2" class="DigNum (strict)"() -> ("Value"=w711:dbl)  [unwired: 2 in, 2 out]
              }
            }
            n507 = property on="UnidadesF" class="Ring (strict)"("Value"=w694) -> ()  [unwired: 2 in, 2 out]
            n508 = Index Array(array=w708, index=w694) -> (element=w709:dbl)
            n509 = property on="PerCentPrecarga" class="DigNum (strict)"() -> ("Value"=w690:sgl)  [unwired: 2 in, 2 out]
            n510 = Multiply(x=w704, y=w709) -> (x*y=w700:dbl)
            n511 = Multiply(x=w700, y=w690) -> (x*y=w703:dbl)
            n512 = Divide(x=w703, y=100.0) -> (x/y=w701:dbl)
            n513 = property on="Valor de control sobrecarga" class="DigNum (strict)"("Value"=w700) -> ()  [unwired: 2 in, 2 out]
            n514 = property on="ArraiUnitats" class="Arr (strict)"() -> ("Value"=w699:cluster{"String":string, "Value":u16}[])  [unwired: 2 in, 2 out]
            n515 = property on="ValorPrecarga" class="DigNum (strict)"("Value"=w701) -> ()  [unwired: 2 in, 2 out]
            n516 = Index Array(array=w699, index=w694) -> (element=w698:cluster{"String":string, "Value":u16})
            n517 = Unbundle By Name(w698) -> ("String"=w695:string)
            n518 = property on="Fuerza" class="DigNum (strict)"() -> ("Caption.Text"=w689:string)  [unwired: 2 in, 2 out]
            n519 = Concatenate Strings(w689, " - " ("string"), w695) -> (w697:string)
            n520 = property class="XYGraph (strict)"("YScale.NameLbl.Text"=w697) -> ()  [unwired: 2 in, 2 out]
          }
          event "UnidadesD": Value Change {
            n521 = event-data() -> ("NewVal"=w717:u16)  [unwired: 1 in, 5 out]
            n522 = property class="DigNum (strict)"(reference=w722, "Value"=sgl 0.0) -> ()  [unwired: 1 in, 2 out]
            n523 = property on="UnidadesD" class="Ring (strict)"() -> ("StringsAndValues[]"=w718:T6)  [unwired: 2 in, 2 out]
            n524 = property class="XYGraph (strict)"() -> ("XScale.NameLbl.Text"=w720:string)  [unwired: 2 in, 2 out]
            n525 = Index Array(array=w718, index=w717) -> (element=w715:cluster{"String":string, "Value":u16})
            n526 = Unbundle By Name(w715) -> ("String"=w713:string)
            n527 = Match Pattern(string=w720, regular expression="-") -> (before substring=w716:string)  [unwired: 1 in, 3 out]
            n528 = Concatenate Strings(w716, "- " ("regular expression"), w713) -> (w714:string)
            n529 = property class="XYGraph (strict)"("XScale.NameLbl.Text"=w714) -> ()  [unwired: 2 in, 2 out]
          }
          event "CaptadorF": Value Change {
            n530 = event-data() -> ()  [unwired: 1 in, 6 out]
            n531 = property class="Ring (strict)"(reference=w725) -> ("Strings []"=w727:string[], "RingText.Text"=w726:string)  [unwired: 1 in, 2 out]
            n532 = Search 1D Array(1D array=w727, element=w726) -> (index of element=w724:i32)  [unwired: 1 in]
            n533 = Equal?(x=w724, y=0) -> (x = y?=w728:bool)
            n534 = flat-sequence {
              tunnel: w729 -> [w741]
              tunnel: w728 -> [w740]
              frame #0 {
                n535 = case shown="True" w740 {
                  tunnel: [w747 w749] -> w733
                  tunnel: [w748 w751] -> w736
                  tunnel: [1 ("index") 0 ("index")] -> w739
                  frame False {
                    n536 = property on="ValorSobrecargaC2" class="DigNum (strict)"() -> ("Value"=w748:dbl)  [unwired: 2 in, 2 out]
                    n537 = property on="UnidadesF_C2" class="Ring (strict)"() -> ("StringsAndValues[]"=w747:T6)  [unwired: 2 in, 2 out]
                  }
                  frame True {
                    n538 = property on="UnidadesF_C1" class="Ring (strict)"() -> ("StringsAndValues[]"=w749:T6)  [unwired: 2 in, 2 out]
                    n539 = property on="ValorSobrecargaC1" class="DigNum (strict)"() -> ("Value"=w751:dbl)  [unwired: 2 in, 2 out]
                  }
                }
                n540 = property on="ConversioUnitatsF" class="Arr (strict)"() -> ("Value"=w744:dbl[])  [unwired: 2 in, 2 out]
                n541 = property on="Calibratge" class="Arr (strict)"() -> ("Value"=w745:dbl[])  [unwired: 2 in, 2 out]
                n542 = Index Array(array=w745, index=w739) -> (element=w743:dbl)
                n543 = Multiply(x=w744, y=w743) -> (x*y=w742:dbl[])
                n544 = property class="Arr (strict)"(reference=w741, "Value"=w742) -> ()  [unwired: 1 in, 2 out]
                n545 = Index Array(array=w733, index=0) -> (element=w731:cluster{"String":string, "Value":u16})
                n546 = Unbundle By Name(w731) -> ("Value"=w730:u16)
                n547 = property on="PerCentPrecarga" class="DigNum (strict)"() -> ("Value"=w734:sgl)  [unwired: 2 in, 2 out]
                n548 = property on="Valor de control sobrecarga" class="DigNum (strict)"("Value"=w736) -> ()  [unwired: 2 in, 2 out]
                n549 = property on="UnidadesF" class="Ring (strict)"("StringsAndValues[]"=w733, "Val(Sgnl)"=w730) -> ()  [unwired: 2 in, 2 out]
                n550 = Multiply(x=w736, y=w734) -> (x*y=w738:dbl)
                n551 = Divide(x=w738, y=100.0) -> (x/y=w735:dbl)
                n552 = property on="ValorPrecarga" class="DigNum (strict)"("Value"=w735) -> ()  [unwired: 2 in, 2 out]
              }
            }
          }
          event "PerCentPrecarga": Value Change {
            n553 = event-data() -> ("NewVal"=w754:sgl)  [unwired: 1 in, 5 out]
            n554 = property on="Valor de control sobrecarga" class="DigNum (strict)"() -> ("Value"=w753:dbl)  [unwired: 2 in, 2 out]
            n555 = Multiply(x=w753, y=w754) -> (x*y=w756:dbl)
            n556 = Divide(x=w756, y=100.0) -> (x/y=w752:dbl)
            n557 = property on="ValorPrecarga" class="DigNum (strict)"("Value"=w752) -> ()  [unwired: 2 in, 2 out]
          }
          event "CaptadorD": Value Change {
            n558 = event-data() -> ("NewVal"=w765:u16)  [unwired: 1 in, 5 out]
            n559 = property on="Calibratge D" class="Arr (strict)"() -> ("Value"=w767:dbl[])  [unwired: 2 in, 2 out]
            n560 = property on="ConversioUnitatsD" class="Arr (strict)"() -> ("Value"=w768:dbl[])  [unwired: 2 in, 2 out]
            n561 = Index Array(array=w767, index=w765) -> (element=w772:dbl)
            n562 = Multiply(x=w768, y=w772) -> (x*y=w771:dbl[])
            n563 = property on="UnidadesD" class="Ring (strict)"() -> ("Value"=w763:u16, "StringsAndValues[]"=w762:T6)  [unwired: 2 in, 2 out]
            n564 = property on="CaptadorD" class="Ring (strict)"() -> ("StringsAndValues[]"=w766:T6)  [unwired: 2 in, 2 out]
            n565 = property class="Arr (strict)"(reference=w769, "Value"=w771) -> ()  [unwired: 1 in, 2 out]
            n566 = Index Array(array=w766, index=w765) -> (element=w764:cluster{"String":string, "Value":u16})
            n567 = Index Array(array=w762, index=w763) -> (element=w761:cluster{"String":string, "Value":u16})
            n568 = Unbundle By Name(w764) -> ("String"=w759:string)
            n569 = Unbundle By Name(w761) -> ("String"=w757:string)
            n570 = Concatenate Strings(w759, " - " ("string"), w757) -> (w760:string)
            n571 = property class="XYGraph (strict)"("XScale.NameLbl.Text"=w760) -> ()  [unwired: 2 in, 2 out]
          }
          event "Paro Emergencia", "Sobrecarga": Value Change {
            n572 = event-data() -> ("NewVal"=w777:bool)  [unwired: 1 in, 5 out]
            n573 = property on="StringsEstatMáquina" class="Arr (strict)"() -> ("Value"=w774:string[])  [unwired: 2 in, 2 out]
            n574 = property on="CodiAturada" class="DigNum (strict)"() -> ("Value"=w773:u32)  [unwired: 2 in, 2 out]
            n575 = case shown="True" w777 {
              tunnel: [w779 w783] -> w775
              tunnel: w776 -> [_ w788]
              tunnel: w774 -> [w780 w782]
              tunnel: w773 -> [w778 w781]
              frame False {
                n576 = Index Array(array=w780, index=w778) -> (element=w779:string)
              }
              frame True {
                n577 = property on="ParoProcessat" class="Bool (strict)"(reference=w788, "Value"=TRUE) -> ()  [unwired: 1 in, 2 out]
                n578 = property on="Procesa datos" class="Bool (strict)"("Value"=FALSE ("Procesa datos")) -> (error out=w786:errorcluster)  [unwired: 2 in, 1 out]
                n579 = property on="Iniciar / Finalizar" class="Bool (strict)"() -> ("Value"=w784:bool)  [unwired: 2 in, 2 out]
                n580 = Index Array(array=w782, index=w781) -> (element=w783:string)
                n581 = case shown="True" w784 {
                  tunnel: w786 -> [_ w790]
                  frame False {
                  }
                  frame True {
                    n582 = property on="Iniciar / Finalizar" class="Bool (strict)"(error in=w790, "Val(Sgnl)"=FALSE ("Value (Signaling)")) -> ()  [unwired: 1 in, 2 out]
                  }
                }
              }
            }
            n583 = property on="Estado ensayo:" class="Str"("Value"=w775) -> ()  [unwired: 2 in, 2 out]
          }
          event "BtTaraD": Value Change {
            n584 = event-data() -> ()  [unwired: 1 in, 6 out]
            n585 = property class="DigNum (strict)"(reference=w794) -> (error out=w793:errorcluster, "Value"=w792:sgl)  [unwired: 1 in, 1 out]
            n586 = property class="DigNum (strict)"(reference=w791, error in=w793, "Value"=w792) -> ()  [unwired: 2 out]
          }
          event "BtTaraF": Value Change {
            n587 = event-data() -> ()  [unwired: 1 in, 6 out]
            n588 = property class="DigNum (strict)"(reference=w797) -> ("Value"=w795:sgl)  [unwired: 1 in, 2 out]
            n589 = property class="DigNum (strict)"(reference=w796, "Value"=w795) -> ()  [unwired: 1 in, 2 out]
          }
          event "PrecargaOn": Value Change {
            n590 = event-data() -> ("NewVal"=w802:bool)  [unwired: 1 in, 5 out]
            n591 = case shown="True" w802 {
              tunnel: w801 -> [_ w806]
              tunnel: w800 -> [_ w804]
              tunnel: w799 -> [_ _]
              tunnel: w798 -> [_ _]
              frame False {
              }
              frame True {
                n592 = property class="DigNum (strict)"(reference=w806) -> (error out=w805:errorcluster, "Value"=w803:sgl)  [unwired: 1 in, 1 out]
                n593 = property class="DigNum (strict)"(reference=w804, error in=w805, "Value"=w803) -> ()  [unwired: 2 out]
              }
            }
          }
        }
        n594 = property on="Stop" class="Bool (strict)"() -> ("Value"=w519:bool)  [unwired: 2 in, 2 out]
      }
      n595 = call <vilib>:"DAQmx Stop Task.vi"("task/channels in"=w232, "error in"=w233) -> ("task out"=w235:refnum<k21>, "error out"=w234:errorcluster)  [unwired: 12 in]
      n596 = call <vilib>:"DAQmx Stop Task.vi"("task/channels in"=w240, "error in"=w239) -> ("task out"=w242:refnum<k21>, "error out"=w241:errorcluster)  [unwired: 12 in]
      n597 = call <vilib>:"DAQmx Clear Task.vi"("task in"=w235, "error in"=w234) -> ()  [unwired: 13 in, 1 out]
      n598 = call <vilib>:"DAQmx Clear Task.vi"("task in"=w242, "error in"=w241) -> ()  [unwired: 13 in, 1 out]
      n599 = control-ref of="Pujar"() -> (w212:refnum<vi>)
      n600 = control-ref of="Salir"() -> (w247:refnum<vi>)
      n601 = control-ref of="Velocidad Ensayo"() -> (w197:refnum<vi>)
      n602 = control-ref of="Velocidad Retorno"() -> (w196:refnum<vi>)
      n603 = control-ref of="VelocitatMàxima"() -> (w217:refnum<vi>)
      n604 = control-ref of="Baixar"() -> (w211:refnum<vi>)
      n605 = control-ref of="MotorBipolar"() -> (w210:refnum<vi>)
      n606 = control-ref of="Active_motor"() -> (w215:refnum<vi>)
      n607 = control-ref of="start"() -> (w213:refnum<vi>)
      n608 = call "SortidaDigitalUSB.vi"(0:w197, 1:w215, 2:w210, 5:w247, 7:w212, 9:w211, 11:w196, 12:w217, 13:w213) -> ()  [unwired: 7 in]
      n609 = Unregister For Events(event registration refnum=w222) -> ()  [unwired: 1 in, 1 out]
      n610 = Current VI's Menubar() -> (w273:refnum<k9>)
      n611 = Delete Menu Items(9:w273) -> (3:w272:refnum<k9>)  [unwired: 3 in, 1 out]
      n612 = Insert Menu Items(8:string[] ["Calibra", "About"] ("item names"), 9:w272) -> (3:w219:refnum<k9>)  [unwired: 4 in, 2 out]
      n613 = while {
        tunnel: w219 -> [w416]
        stop <- w415 stop-if-true
        n614 = Get Menu Selection(0:w416, 1:200 ("ms timeout (200)")) -> (6:w417:string)  [unwired: 2 in, 4 out]
        n615 = case shown="\"Calibra\"" w417 {
          frame "About" {
            n616 = call "About.vi"() -> ()  [unwired: 1 in]
          }
          frame "Calibra" {
            n617 = control-ref of="Password"() -> (w421:refnum<vi>)
            n618 = property class="Str"(reference=w421) -> ("Value"=w420:string)  [unwired: 1 in, 2 out]
            n619 = call "Password.vi"() -> ("Password"=w422:string)  [unwired: 17 in, 2 out]
            n620 = Equal?(x=w420, y=w422) -> (x = y?=w419:bool)
            n621 = case shown="True" w419 {
              frame False {
              }
              frame True {
                n622 = call "Calibratge.vi"() -> ("OK ?"=w423:bool)  [unwired: 10 in]
                n623 = case shown="True" w423 {
                  frame False {
                  }
                  frame True {
                    n624 = control-ref of="Valor de control sobrecarga"() -> (w432:refnum<vi>)
                    n625 = call "ReadCal.vi"() -> ("SobrecargaC2"=w430:dbl, "ResoExten"=w438:i8, "TextExtensometre"=w451:string, "TextDeformacio"=w450:string, "SegonCaptador"=w463:string, "MotorBipolar"=w426:bool, "UnitatsC2"=w474:string, "UnitatsC1"=w476:string, "PrimerCaptador"=w464:string, "ViuMotor"=w424:bool, "ExtenPoten"=w428:bool, "SobrecargaC1"=w431:dbl, "Password"=w489:string, "Pendents"=w444:dbl[], "VelocitatMàxima"=w436:dbl)  [unwired: 4 in, 9 out]
                    n626 = property on="ResoExten" class="Ring (strict)"("Value"=w438) -> ()  [unwired: 2 in, 2 out]
                    n627 = control-ref of="ValorSobrecargaC1"() -> (w435:refnum<vi>)
                    n628 = control-ref of="ValorSobrecargaC2"() -> (w434:refnum<vi>)
                    n629 = Decimal String To Number(string=w463) -> (number=w471:i32)  [unwired: 2 in, 1 out]
                    n630 = property class="DigNum (strict)"(reference=w434, "Value"=w430) -> ()  [unwired: 1 in, 2 out]
                    n631 = Decimal String To Number(string=w464) -> (number=w472:i32)  [unwired: 2 in, 1 out]
                    n632 = control-ref of="ViuMotor"() -> (w425:refnum<vi>)
                    n633 = control-ref of="MotorBipolar"() -> (w427:refnum<vi>)
                    n634 = property on="Células" class="Ring (strict)"() -> ("StringsAndValues[]"=w470:T4)  [unwired: 2 in, 2 out]
                    n635 = property class="DigNum (strict)"(reference=w435, "Value"=w431) -> ()  [unwired: 1 in, 2 out]
                    n636 = control-ref of="ExtenPoten"() -> (w429:refnum<vi>)
                    n637 = property class="Bool (strict)"(reference=w429, "Value"=w428) -> ()  [unwired: 1 in, 2 out]
                    n638 = property class="Bool (strict)"(reference=w425, "Value"=w424) -> ()  [unwired: 1 in, 2 out]
                    n639 = property class="Bool (strict)"(reference=w427, "Value"=w426) -> ()  [unwired: 1 in, 2 out]
                    n640 = property on="CaptadorF" class="Ring (strict)"() -> ("Value"=w433:u16)  [unwired: 2 in, 2 out]
                    n641 = case shown="1" w433 {
                      tunnel: w432 -> [w491 w493]
                      tunnel: w431 -> [w490 _]
                      tunnel: w430 -> [_ w492]
                      frame 0, Default {
                        n642 = property class="DigNum (strict)"(reference=w491, "Value"=w490) -> ()  [unwired: 1 in, 2 out]
                      }
                      frame 1 {
                        n643 = property class="DigNum (strict)"(reference=w493, "Value"=w492) -> ()  [unwired: 1 in, 2 out]
                      }
                    }
                    n644 = control-ref of="ArraiUnitats"() -> (w475:refnum<vi>)
                    n645 = Index Array(array=w470, index=w472) -> (element=w462:cluster{"String":string, "Value":u8})
                    n646 = Index Array(array=w470, index=w471) -> (element=w468:cluster{"String":string, "Value":u8})
                    n647 = control-ref of="Pendents"() -> (w487:refnum<vi>)
                    n648 = Unbundle(w462) -> ("Value"=w461:u8)  [unwired: 1 out]
                    n649 = control-ref of="VelocitatMàxima"() -> (w437:refnum<vi>)
                    n650 = property class="DigNum (strict)"(reference=w437, "Value"=w436) -> ()  [unwired: 1 in, 2 out]
                    n651 = call "UnitatsStringsValors.vi"("UnitatsC1"=w476, "Arr Refnum"=w475) -> ("Array 2"=w466:cluster{"String":string, "Value":u16}[])  [unwired: 1 out]
                    n652 = call "UnitatsStringsValors.vi"("UnitatsC1"=w474, "Arr Refnum"=w475) -> ("Array 2"=w473:cluster{"String":string, "Value":u16}[])  [unwired: 1 out]
                    n653 = property class="Arr (strict)"(reference=w487, "Value"=w444) -> ()  [unwired: 1 in, 2 out]
                    n654 = Index Array(array=w444, index=3) -> (element=w448:dbl)
                    n655 = Unbundle(w468) -> ("Value"=w467:u8)  [unwired: 1 out]
                    n656 = property on="Password" class="Str"("Value"=w489) -> ()  [unwired: 2 in, 2 out]
                    n657 = property on="Celula_0" class="DigNum (strict)"("Value"=w461) -> ()  [unwired: 2 in, 2 out]
                    n658 = property on="UnidadesF_C2" class="Ring (strict)"("StringsAndValues[]"=w473) -> ()  [unwired: 2 in, 2 out]
                    n659 = Equal To 0?(x=w448) -> (x = 0?=w452:bool)
                    n660 = case shown="0, Default" w467 {
                      tunnel: w462 -> [w503 w504]
                      tunnel: w468 -> [w502 _]
                      tunnel: [w501 w505] -> w469
                      frame 0, Default {
                        n661 = Build Array(w503, w502) -> (w501:cluster{"String":string, "Value":u8}[])
                      }
                      frame 17 {
                        n662 = Build Array(w504) -> (w505:cluster{"String":string, "Value":u8}[])
                      }
                    }
                    n663 = case shown="False" w452 {
                      tunnel: w451 -> [w496 _]
                      tunnel: w450 -> [w497 w500]
                      tunnel: [w495 w499] -> w447
                      tunnel: [TRUE ("Extensometre") FALSE ("Extensometre")] -> w441
                      frame False {
                        n664 = Build Array(w497, w496) -> (w495:string[])
                      }
                      frame True {
                        n665 = Build Array(w500) -> (w499:string[])
                      }
                    }
                    n666 = property on="UnidadesF_C1" class="Ring (strict)"("StringsAndValues[]"=w466) -> ("Value"=w465:u16)  [unwired: 2 in, 2 out]
                    n667 = Index Array(array=w444, index=2) -> (element=w480:dbl)
                    n668 = Index Array(array=w444, index=0) -> (element=w481:dbl)
                    n669 = Index Array(array=w444, index=1) -> (element=w455:dbl)
                    n670 = Index Array(array=w444, index=3) -> (element=w454:dbl)
                    n671 = control-ref of="ConversioUnitatsD"() -> (w460:refnum<vi>)
                    n672 = Build Array(w481, w480) -> (w478:dbl[])
                    n673 = control-ref of="Calibratge"() -> (w479:refnum<vi>)
                    n674 = Build Array(w455, w454) -> (w453:dbl[])
                    n675 = control-ref of="ConversioUnitatsF"() -> (w488:refnum<vi>)
                    n676 = property on="Extensometre" class="Bool (strict)"("Value"=w441) -> ()  [unwired: 2 in, 2 out]
                    n677 = control-ref of="Calibratge D"() -> (w458:refnum<vi>)
                    n678 = property class="Arr (strict)"(reference=w460) -> ("Value"=w445:dbl[])  [unwired: 1 in, 2 out]
                    n679 = property class="Arr (strict)"(reference=w479, "Value"=w478) -> ()  [unwired: 1 in, 2 out]
                    n680 = property on="UnidadesF" class="Ring (strict)"("StringsAndValues[]"=w466, "Value"=w465) -> ()  [unwired: 2 in, 2 out]
                    n681 = property class="Arr (strict)"(reference=w458, "Value"=w453) -> ()  [unwired: 1 in, 2 out]
                    n682 = property class="Arr (strict)"(reference=w488) -> ("Value"=w486:dbl[])  [unwired: 1 in, 2 out]
                    n683 = Index Array(array=w444, index=0) -> (element=w477:dbl)
                    n684 = property on="CaptadorD" class="Ring (strict)"("Strings []"=w447, "Value"=0 ("index")) -> ()  [unwired: 2 in, 2 out]
                    n685 = Index Array(array=w444, index=1) -> (element=w443:dbl)
                    n686 = property on="CaptadorF" class="Ring (strict)"("StringsAndValues[]"=w469, "Value"=w461) -> ()  [unwired: 2 in, 2 out]
                    n687 = Multiply(x=w486, y=w477) -> (x*y=w484:dbl[])
                    n688 = control-ref of="FactorsUnitatsPendents_F"() -> (w485:refnum<vi>)
                    n689 = Multiply(x=w445, y=w443) -> (x*y=w442:dbl[])
                    n690 = control-ref of="FactorsUnitatsPendents_D"() -> (w459:refnum<vi>)
                    n691 = property class="Arr (strict)"(reference=w485, "Value"=w484) -> ()  [unwired: 1 in, 2 out]
                    n692 = property class="Arr (strict)"(reference=w459, "Value"=w442) -> ()  [unwired: 1 in, 2 out]
                  }
                }
              }
            }
          }
          frame Default {
          }
        }
        n693 = property on="Stop" class="Bool (strict)"() -> ("Value"=w415:bool)  [unwired: 2 in, 2 out]
      }
    }
    frame #5 {
      n694 = property on="rings" class="Arr (strict)"() -> ("Value"=w1112:refnum<vi>[])  [unwired: 2 in, 2 out]
      n695 = call "GuardaValorsPantalla.vi"("Rings"=w1112) -> ()  [unwired: 9 in, 1 out]
    }
    frame #6 {
      n696 = Quit LabVIEW(quit? (T)=TRUE) -> ()
    }
  }
